vi "TLB Native Dynamic Events ver 0.13a.vi"() -> ()   [LabVIEW 2018]
uses:
  Labview Training Phase 2/Enum Controls/States for Action Engine.ctl
  TLB Type Definitions/State Type Definitions, for 0.26g versions and later 2.ctl
  TLB Type Definitions/Intruction Type Definitions.ctl
  TLB Type Definitions/Encoder cluster.ctl
  Experimental VI's/Archived VI's/MOTOR CONTROL NO PID Type Def.ctl
  Underlying VI's/I2C Master VI/I2C MASTER Type Def.ctl
  TLB Type Definitions/PING CLUSTER.ctl
  <vilib>/Studica/Studica Toolkit/NavX/NavX.lvlib
  <vilib>/Studica/Studica Toolkit/Background/DIO Channel.ctl
  Underlying VI's/NavX VI/navX type def.ctl
  <vilib>/myRIO/Instrument Drivers/Utilities/Utilities.lvlib
  <vilib>/Studica/Studica Toolkit/Background/I2C Channel.ctl
  Underlying VI's/I2C Master VI/I2C_MASTER_WRITE_NEW Type Def.ctl
  <vilib>/userdefined/High Color/IMAQdx.ctl
  Underlying VI's/Webcam FGV Low level ver/State control.ctl
  TLB Type Definitions/Vision cluster.ctl
  <vilib>/NI_Real-Time Target Support.lvlib
  <vilib>/Studica/Studica Toolkit/NavX/TypeDefs/Flags/Z900_navX_Flags_CalibrationStatusTypeDef.ctl
  <vilib>/Studica/Studica Toolkit/NavX/TypeDefs/Flags/Z900_navX_Flags_OpStatusTypeDef.ctl
  <vilib>/Utility/RT CPU Load.ctl
panel:
  out "CPU loads":T1[](array[typedef]) {"ISR (%)" format="%#.2f"; "Idle (%)" format="%#.2f"; "Background (%)" format="%#.2f"; "Normal (%)" format="%#.2f"; "Above Normal (%)" format="%#.2f"; "High (%)" format="%#.2g"; "Timed Structures (%)" format="%#.2g"; "Time Critical (%)" format="%#.2g"; "Total (%)" format="%#.2g"}
  in  "Red LED":bool
  out "Object Center Coordinates":cluster{"x":sgl, "y":sgl}
  out "Object detection cluster":T2
  in  "Mode":enum16{"Ball", "Soap", "Gel", "Pipe", "None"}(ring)
  in  "Latch":bool
  in  "y Stepper value":u8
  out "Arduino Data":T3
  in  "Arduino mode":T4
  out "Detect?":bool
  out "Status":T7 {"OP Status" items=["INITIALIZING", "SELFTEST_IN_PROGRESS", "ERROR", "IMU_AUTOCAL_IN_PROGRESS", "NORMAL"]; "Calibration Status" items=["IMU_CAL_STATE_MASK"=3, "IMU_CAL_STATE_INPROGRESS"=0, "IMU_CAL_STATE_ACCUMULATE"=1, "IMU_CAL_STATE_COMPLETE"=2]}
  out "NavX Readings":T8
  out "TASK ENABLE":bool
  out "Rising Edge":bool
  in  "Green LED":bool
  out "Task Selection":u8
  out "Object detected?":bool
  out "I2C Error":errorcluster
  out "Speed & distance":T9
  out "State Logic":T10=enum."Startup"
  out "elements":T11[](array[typedef])
  in  "STOP TASK":bool
  in  "OK Button":bool
  in  "STOP":bool
  out "error out":errorcluster
  out "Action Queue Items":i32
  out "State Logic Queue Items":i32
  out "Action Queues items":string[](array[string])=["Hardware reset", "Software reset", ""]
  out "Action State":string
  # "TLB FRAMEWORK STATUS"
  # "System Health Status Update"
  # "Test Programme written by Calvin Loke    Dated: 28 Aug 2019\nTest Programme revised by Dr Alex See   Dated 30 Aug 2019\n\nProgramme version:   TLB Native Dynamic Events ver 0.04b.vi"
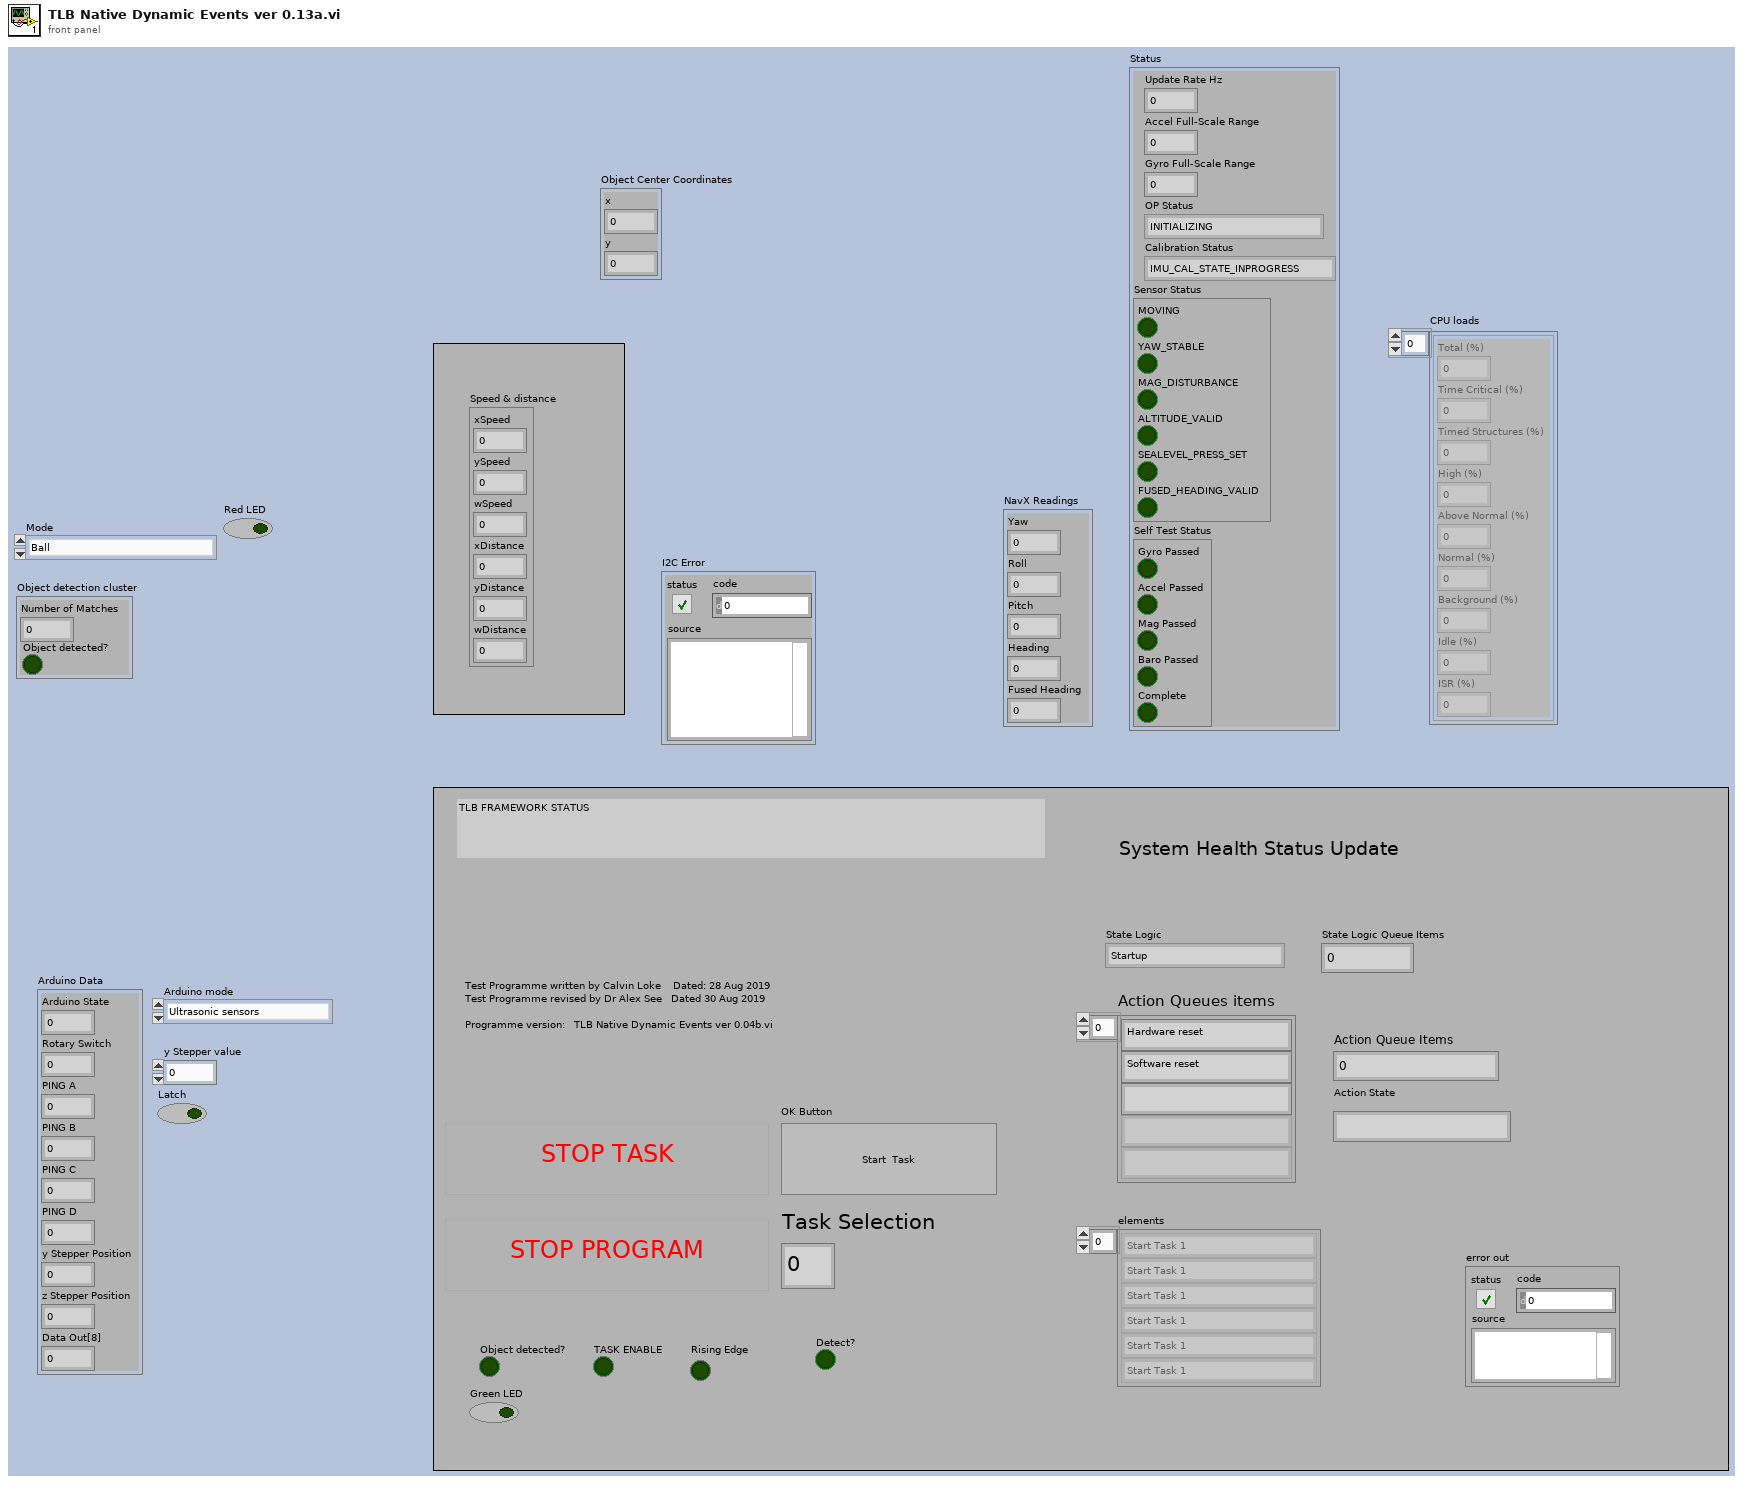
[diagram p1: front panel]
types:
  T1 = typedef "NI_Real-Time Target Support.lvlib/RT CPU Load.ctl" = cluster{"Total (%)":dbl, "Time Critical (%)":dbl, "Timed Structures (%)":dbl, "High (%)":dbl, "Above Normal (%)":dbl, "Normal (%)":dbl, "Background (%)":dbl, "Idle (%)":dbl, "ISR (%)":dbl}
  T2 = cluster{"Number of Matches":i32, "Object detected?":bool}
  T3 = cluster{"Arduino State":u8, "Rotary Switch":u8, "PING A":u8, "PING B":u8, "PING C":u8, "PING D":u8, "y Stepper Position":u8, "z Stepper Position":u8, "Data Out[8]":u8}
  T4 = typedef "I2C_MASTER_WRITE_NEW Type Def.ctl" = enum16{"Ultrasonic sensors", "Stepper origin", "zStepper 13.3k", "zStepper 13k", "zStepper 12k", "zStepper 11k", "zStepper 10k", "zStepper 9k", "zStepper 8k", "zStepper 7k", "zStepper 6k", "zStepper 5k", "zStepper 4k", "zStepper 3k", "zStepper 2k", "zStepper 1k", "zStepper 900", "zStepper 800", "zStepper 700", "zStepper 600", "zStepper 500", "zStepper 400", "zStepper 300", "zStepper 200", "zStepper 100", "zStepper 0", "yStepper control", "Open Claw", "Close Claw", "Soft Reset"}
  T5 = typedef "NavX.lvlib/Z900_navX_Flags_OpStatusTypeDef.ctl" = u8
  T6 = typedef "NavX.lvlib/Z900_navX_Flags_CalibrationStatusTypeDef.ctl" = u8
  T7 = cluster{"Update Rate Hz":u8, "Accel Full-Scale Range":u8, "Gyro Full-Scale Range":u16, "OP Status":T5, "Calibration Status":T6, "Sensor Status":cluster{"MOVING":bool, "YAW_STABLE":bool, "MAG_DISTURBANCE":bool, "ALTITUDE_VALID":bool, "SEALEVEL_PRESS_SET":bool, "FUSED_HEADING_VALID":bool}, "Self Test Status":cluster{"Gyro Passed":bool, "Accel Passed":bool, "Mag Passed":bool, "Baro Passed":bool, "Complete":bool}}
  T8 = cluster{"Yaw":dbl, "Roll":dbl, "Pitch":dbl, "Heading":dbl, "Fused Heading":dbl}
  T9 = cluster{"xSpeed":dbl, "ySpeed":dbl, "wSpeed":dbl, "xDistance":dbl, "yDistance":dbl, "wDistance":dbl}
  T10 = typedef "State Type Definitions, for 0.26g versions and later 2.ctl" = enum16{"None", "Startup", "Move to Angle", "True Stop", "Idle", "Shutdown", "Task 1A", "Task 1B", "Task 2:Raise Arm", "Task 2:Sensor Mode", "Task 2:Reverse Mode", "Task 3", "Task 4_A", "Task 4_B", "Task 4_C", "Task 4_D", "Task 5A", "Task 5B", "Task 5C", "Task 5D", "Task 5E: POSITION ARM", "Task 5F: ARM GRAB HEIGHT", "Task 5G: CLOSE CLAW", "Task 5H: RAISE ARM", "Task 6_A", "Task 6_B", "Task 7", "Task 8A: RAISE ARM", "Task 8B: MOVE TO BOX", "Task 8C: CAM BURST", "Task 8D: PROCESS IMAGE", "Task 8E: ROBOT ADJUST", "Task 8F: CAM BURST 2", "Task 8G: PROCESS IMAGE 2", "Task 8H: ARM ADJUST", "Task 8I: ARM GRAB HEIGHT", "Task 8J: CLOSE CLAW", "Task 8K: RAISE MY SWORD", "Task 9A: Raise Arm", "Task 9B: Rotate to Angle", "Task 9C: Detect Box", "Task 9D: MOVE FORWARD", "Task 9E: MOVE LEFT", "Task 9F: SCAN BOX", "Task 9G: MOVE RIGHT", "Task 9H: SCAN BOX 2", "Task 9I: ROTATE 90 CW", "Task 9J: FORWARD", "Task 9K: MOVE RIGHT", "Task 9L: SCAN BOX 3", "Task 9M: MOVE RIGHT", "Task 9N: SCAN BOX 4", "PENIS", "PENIS 2", "PENIS 3", "Task 9R: PROCESS COLOUR", "Task A1: Task 9 Open cam", "Task A2: Task 9 Move Arm", "Task A3: Task 9 Set Timer", "Task A4: Tasl 9 Capture images", "Task A5: Task 9 Close camera", "Task A6: Process Colour", "Task A7: Dispose Camera Buffer"}
  T11 = typedef "Intruction Type Definitions.ctl" = enum16{"None", "Start Task 1", "Start Task 2", "Start Task 3", "Start Task 4", "Start Task 5", "Start Task 6", "Start Task 7", "Start Task 8 - BALL", "Start Task 8 - Gel", "Start Task 8 - Pipe", "Start Task 8 - Soap", "Start Task 9", "Start Task A", "Start Task B", "Exit"}
  T12 = typedef "States for Action Engine.ctl" = enum16{"Initialize", "Write", "Read"}
  T13 = typedef "DIO Channel.ctl" = enum16{"Not Connected", "A/DIO1", "A/DIO2", "A/DIO3", "A/DIO4", "A/DIO5", "A/DIO6", "A/DIO7", "A/DIO13", "B/DIO1", "B/DIO2", "B/DIO3", "B/DIO4", "B/DIO5", "B/DIO6", "B/DIO7", "B/DIO13", "C/DIO0", "C/DIO1", "C/DIO2", "C/DIO3", "C/DIO4", "C/DIO5", "C/DIO6", "C/DIO7"}
  T14 = typedef "Vision cluster.ctl" = cluster{"Recognized Object":bool, "Object X coordinate":dbl, "Object Y coordinate":dbl}
  T15 = typedef "PING CLUSTER.ctl" = cluster{"PING_A":u8, "PING_B":u8, "PING_C":u8, "PING_D":u8}
  T16 = typedef "Encoder cluster.ctl" = cluster{"xDistance":dbl, "yDistance":dbl, "wDistance":dbl}
  T17 = typedef "I2C Channel.ctl" = enum16{"Not Connected", "A", "B"}
  T18 = typedef "navX type def.ctl" = enum16{"Get i2C reference", "Read Values", "Zero Yaw"}
  T19 = typedef "State Type Definitions.ctl" = enum16{"None", "Startup", "Move to Angle", "True Stop", "Idle", "Shutdown", "Task 1", "Task 2:Raise Arm", "Task 2:Sensor Mode", "Task 2:Reverse Mode", "Task 3", "Task 4_A", "Task 4_B", "Task 4_C", "Task 4_D", "Task 5A: ARM CAM HEIGHT", "Task 5B: MOVE TO BOX", "Task 5C: CAM BURST", "Task 5D: PROCESS IMAGE", "Task 5E: POSITION ARM", "Task 5F: ARM GRAB HEIGHT", "Task 5G: CLOSE CLAW", "Task 5H: RAISE ARM", "Task 6_A", "Task 6_B", "Task 7", "Task 8A: RAISE ARM", "Task 8B: MOVE TO BOX", "Task 8C: CAM BURST", "Task 8D: PROCESS IMAGE", "Task 8E: ROBOT ADJUST", "Task 8F: CAM BURST 2", "Task 8G: PROCESS IMAGE 2", "Task 8H: ARM ADJUST", "Task 8I: ARM GRAB HEIGHT", "Task 8J: CLOSE CLAW", "Task 8K: RAISE MY SWORD", "Task 9A: Raise Arm", "Task 9B: Rotate to Angle", "Task 9C: Detect Box", "Task 9D: MOVE FORWARD", "Task 9E: MOVE LEFT", "Task 9F: SCAN IMAGE", "Task 9G: PROCESS COLOUR", "Task 9H: MOVE RIGHT", "Task 9I: SCAN IMAGE", "Task 9J: PROCESS COLOUR", "Task 9K: ROTATE 90 CW", "Task 9L: MOVE FORWARD", "Task 9M: MOVE RIGHT", "Task 9N: SCAN IMAGE", "Task 9O: PROCESS COLOUR", "Task 9P: MOVE RIGHT", "Task 9Q: SCAN IMAGE", "Task 9R: PROCESS COLOUR"}
  T20 = typedef "State Type Definitions.ctl" = enum16{"None", "Startup", "Move to Angle", "True Stop", "Idle", "Shutdown", "Task 1", "Task 2", "Task 3", "Task 4_A", "Task 4_B", "Task 4_C", "Task 5", "Task 6", "Task 7", "Task 8", "Task 9", "Task A", "Task B"}
  T21 = typedef "MOTOR CONTROL NO PID Type Def.ctl" = enum16{"Init", "Front Back", "Left Right", "Rotate", "Stop", "Latch"}
  T22 = typedef "State control.ctl" = enum16{"Initialise", "Start camera", "Continuous Acquisition ", "Stop camera", "Dispose all"}
  T23 = typedef "IMAQdx.ctl" = refnum<k21>
  T24 = cluster{"DIO Channel":T13, "FPGA VI Reference Out":refnum<k20>}
  T25 = cluster{"I2C Ref Out":cluster{"I2C Channel":T17, "FPGA VI Reference Out":refnum<k20>}, "Connected":bool, "Slave Address (7-bit)":u8, "Registry":u8[]}
  T26 = typedef "IMAQ Image.ctl" = refnum<image>
  T27 = typedef "I2C MASTER Type Def.ctl" = enum16{"Last State", "Mode 0", "Mode 1", "Mode 2", "Mode 3", "Mode 4", "Mode 5", "Mode 6", "Mode 7", "Mode 8", "Mode 9", "Mode 10"}
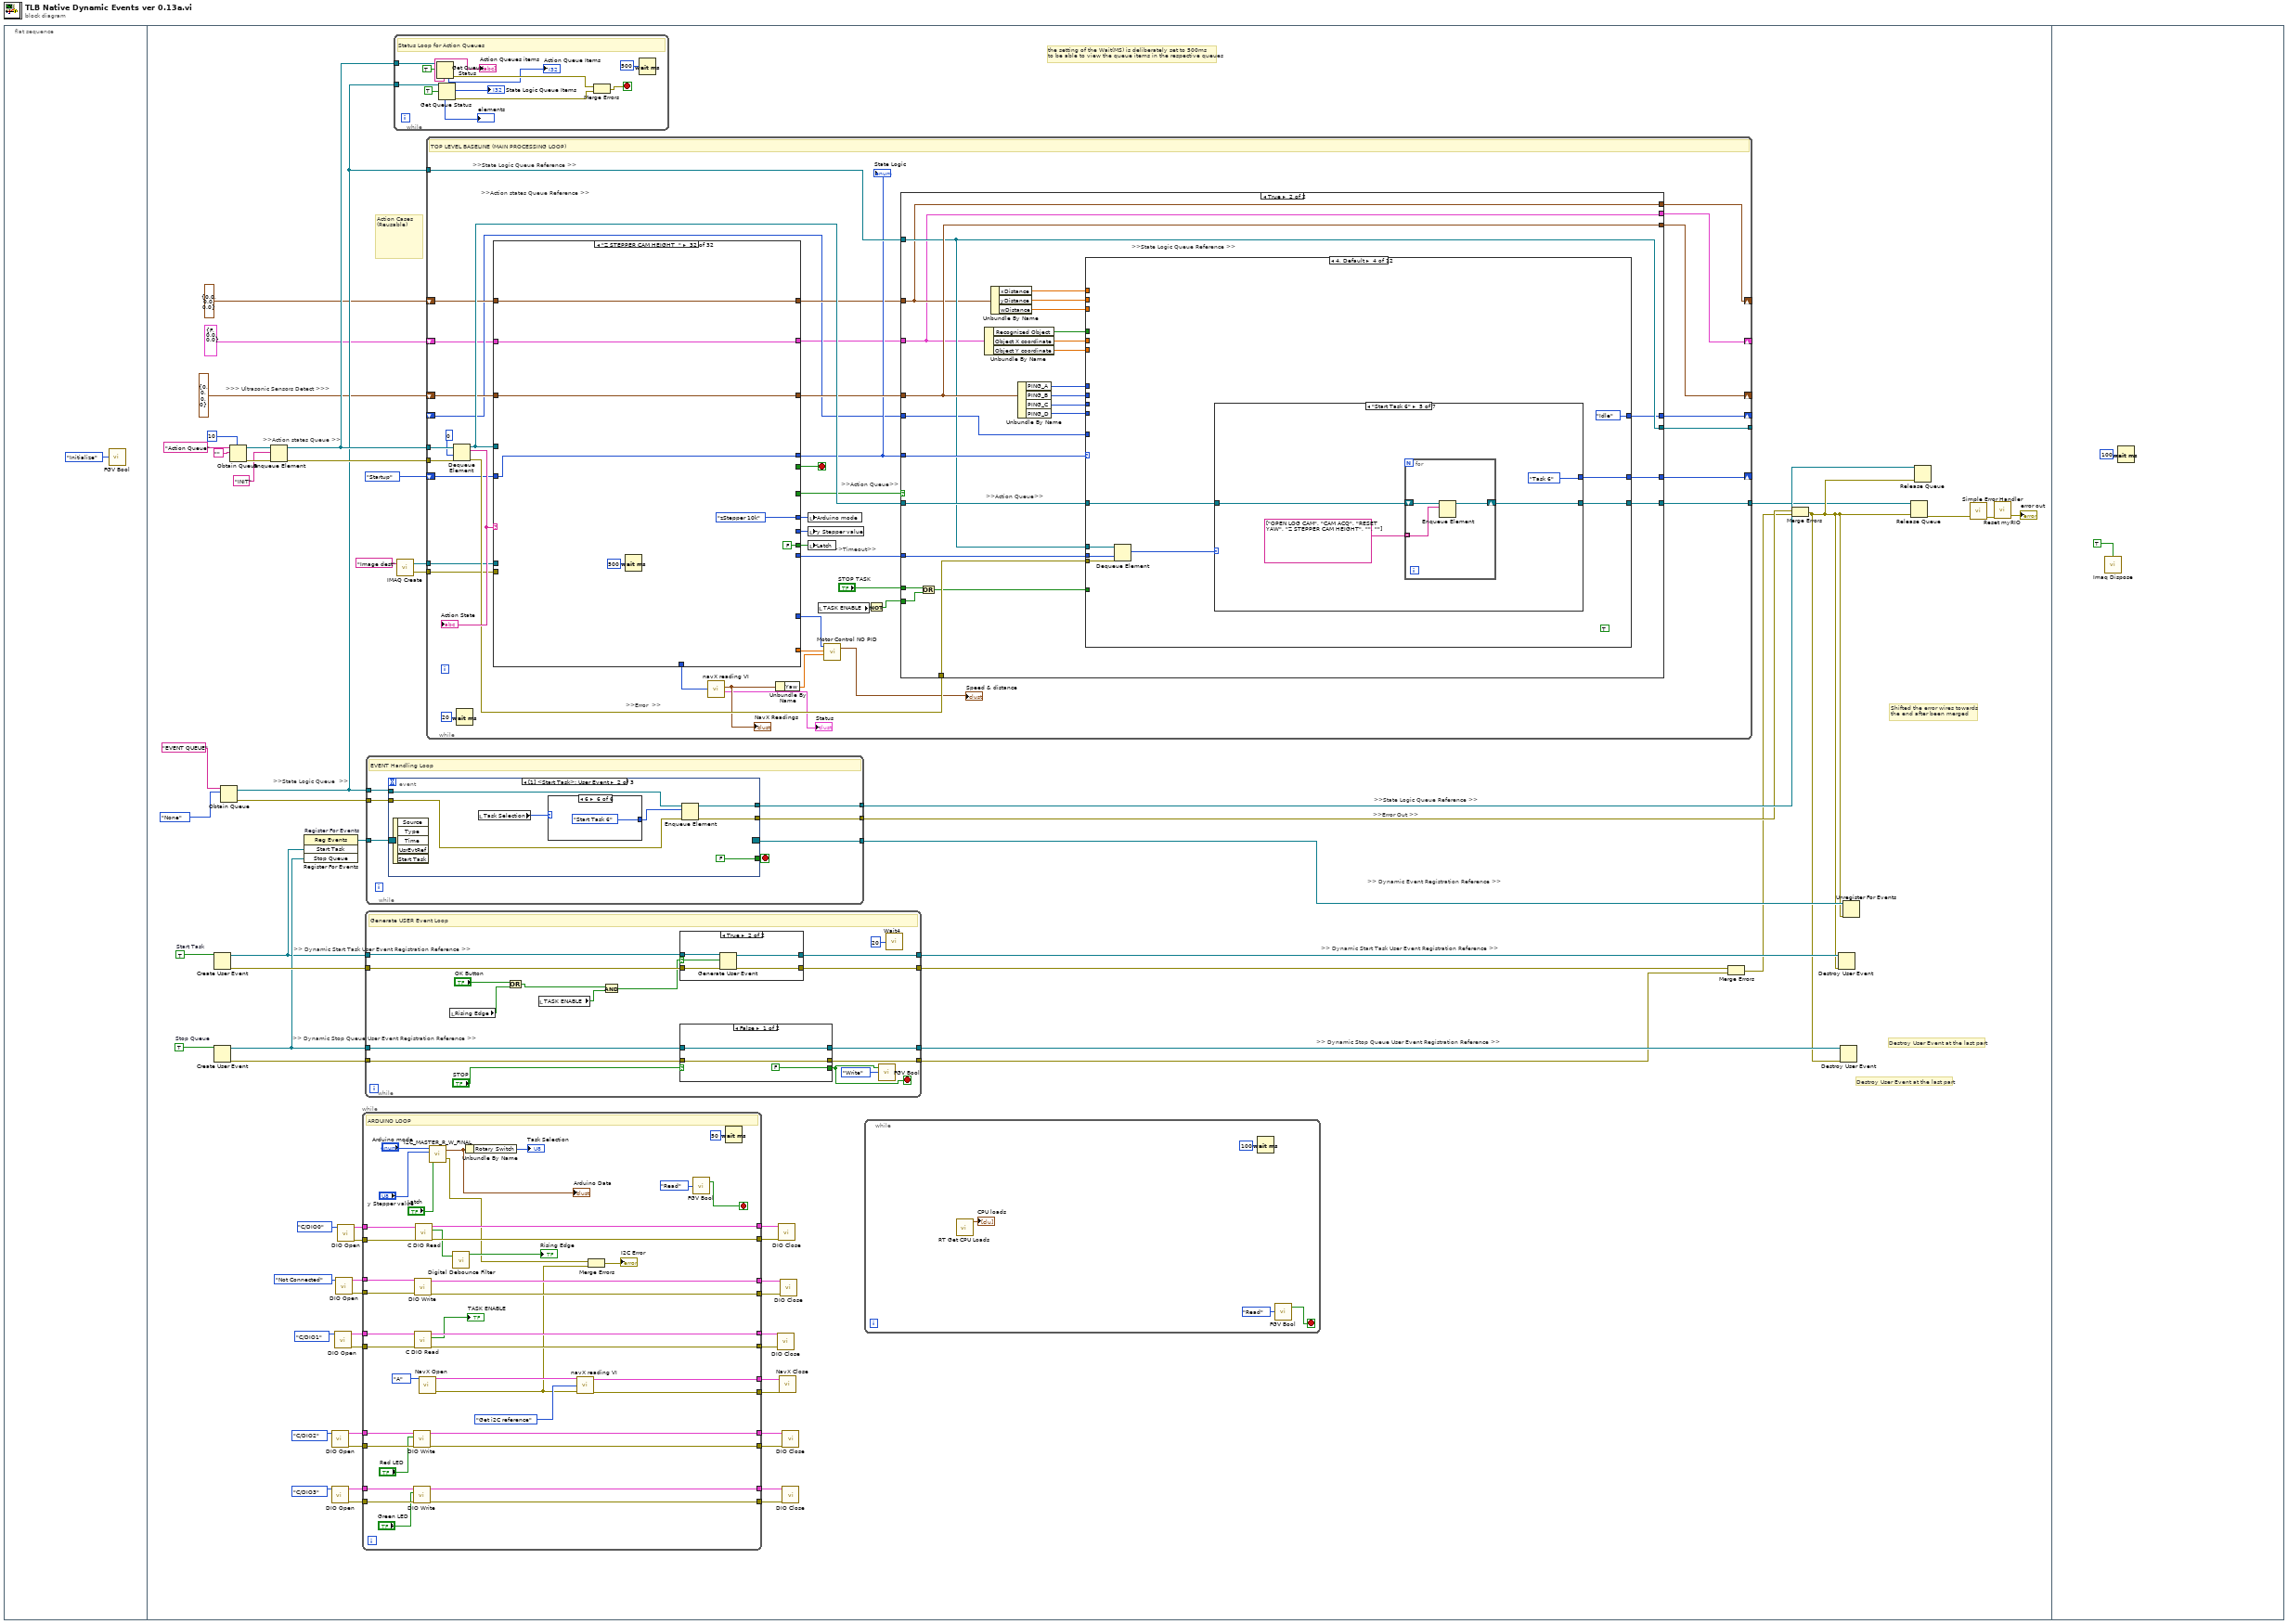
[diagram p0: block diagram]
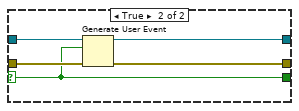
[diagram p2: hidden frame]
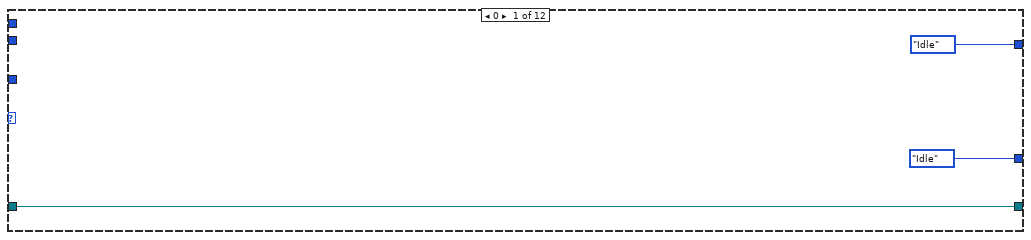
[diagram p5: hidden frame]
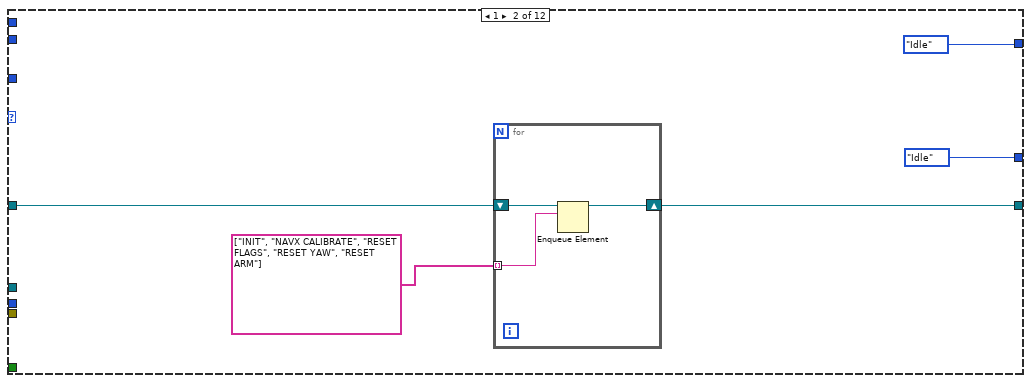
[diagram p6: hidden frame]
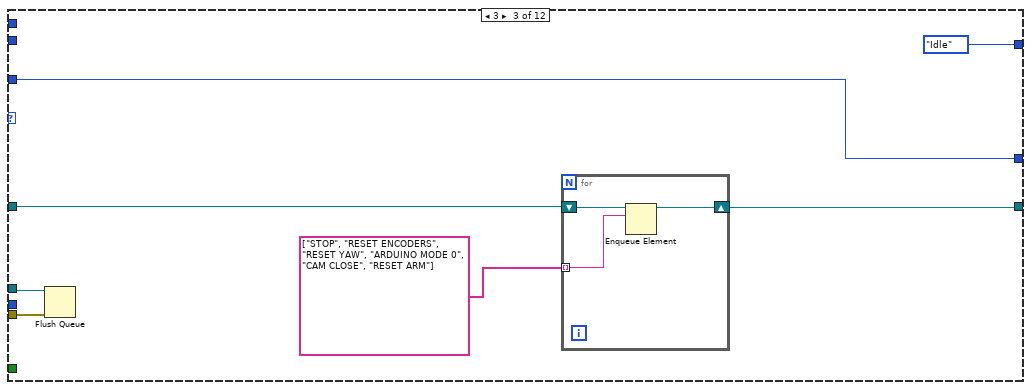
[diagram p7: hidden frame]
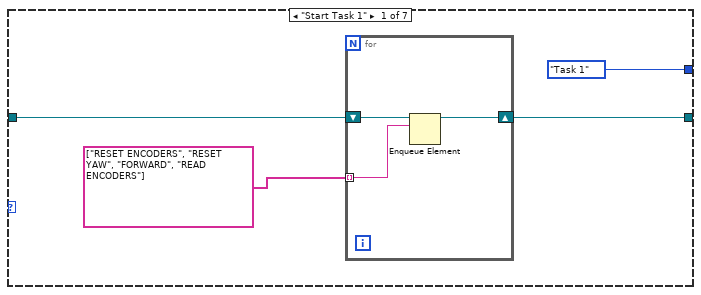
[diagram p8: hidden frame]
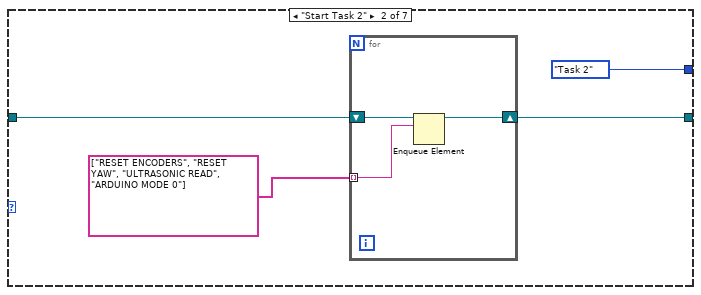
[diagram p9: hidden frame]
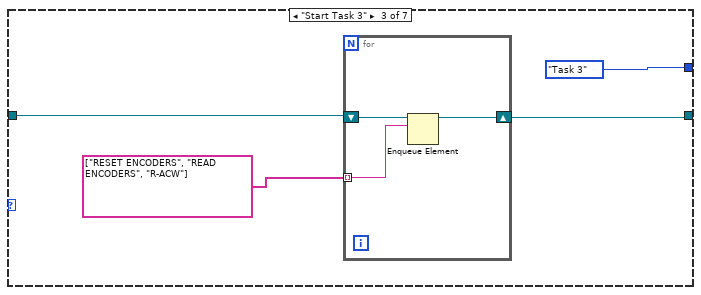
[diagram p10: hidden frame]
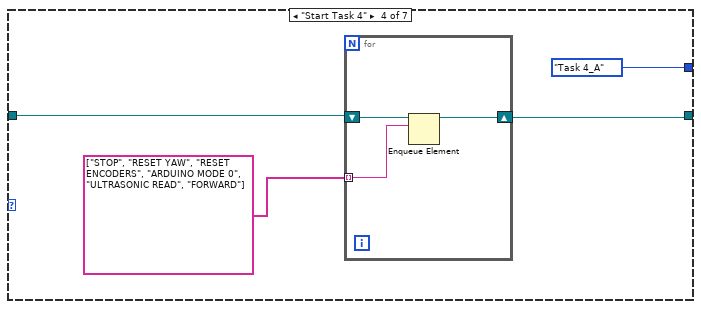
[diagram p11: hidden frame]
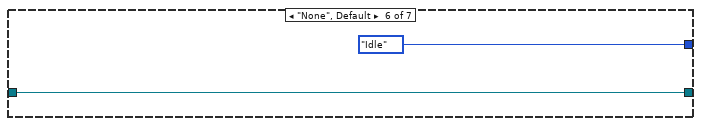
[diagram p12: hidden frame]
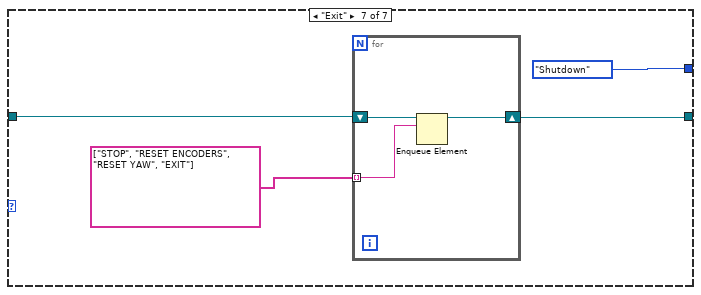
[diagram p13: hidden frame]
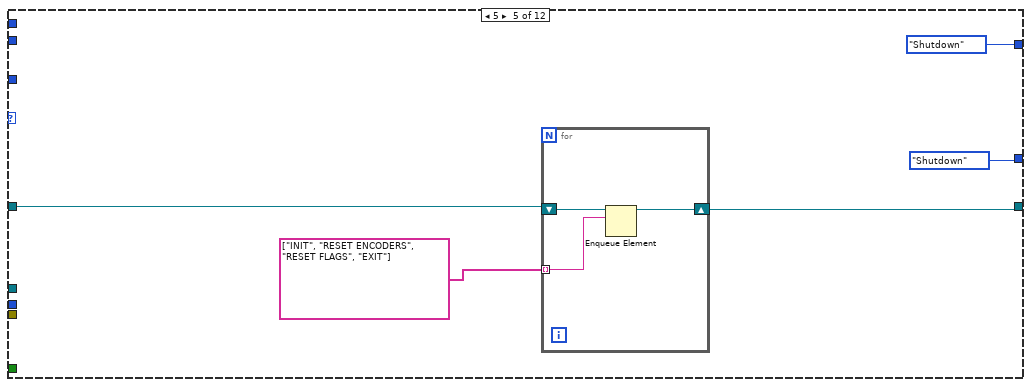
[diagram p14: hidden frame]
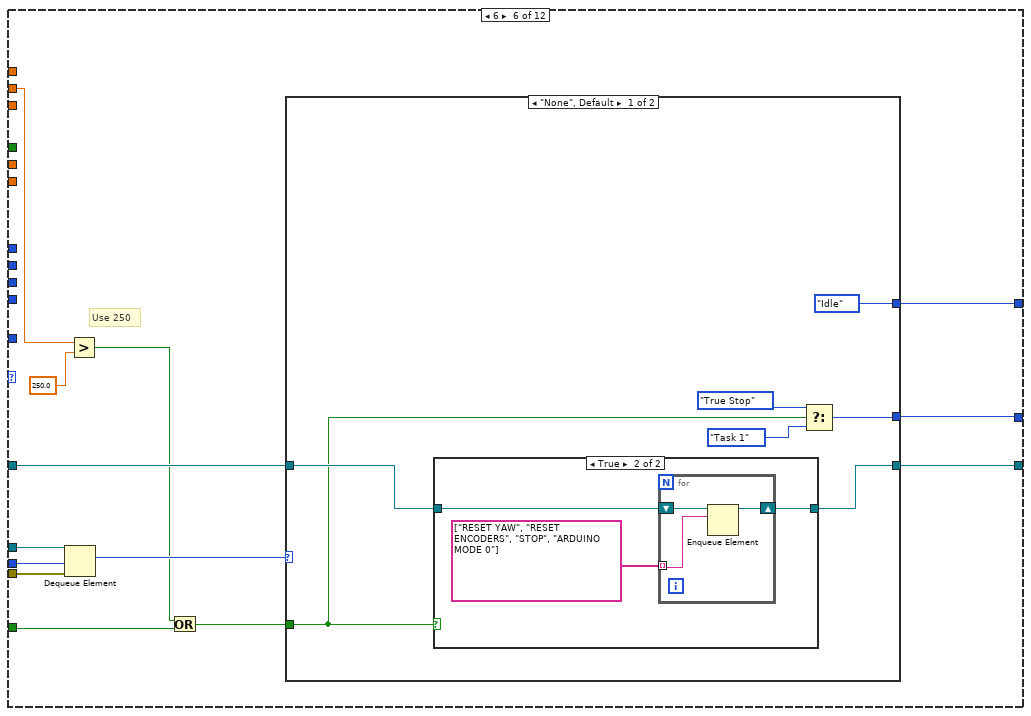
[diagram p15: hidden frame]
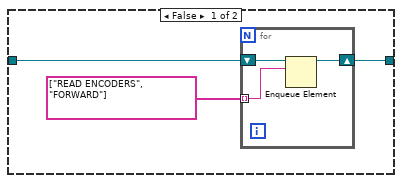
[diagram p16: hidden frame]
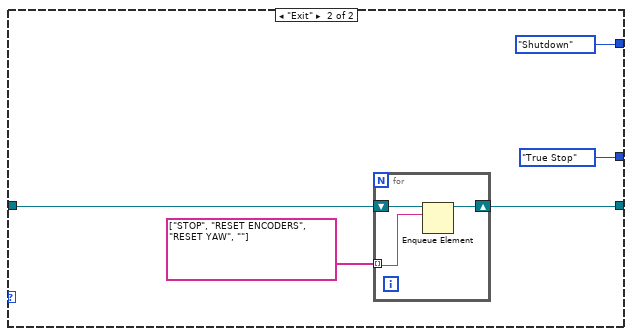
[diagram p17: hidden frame]
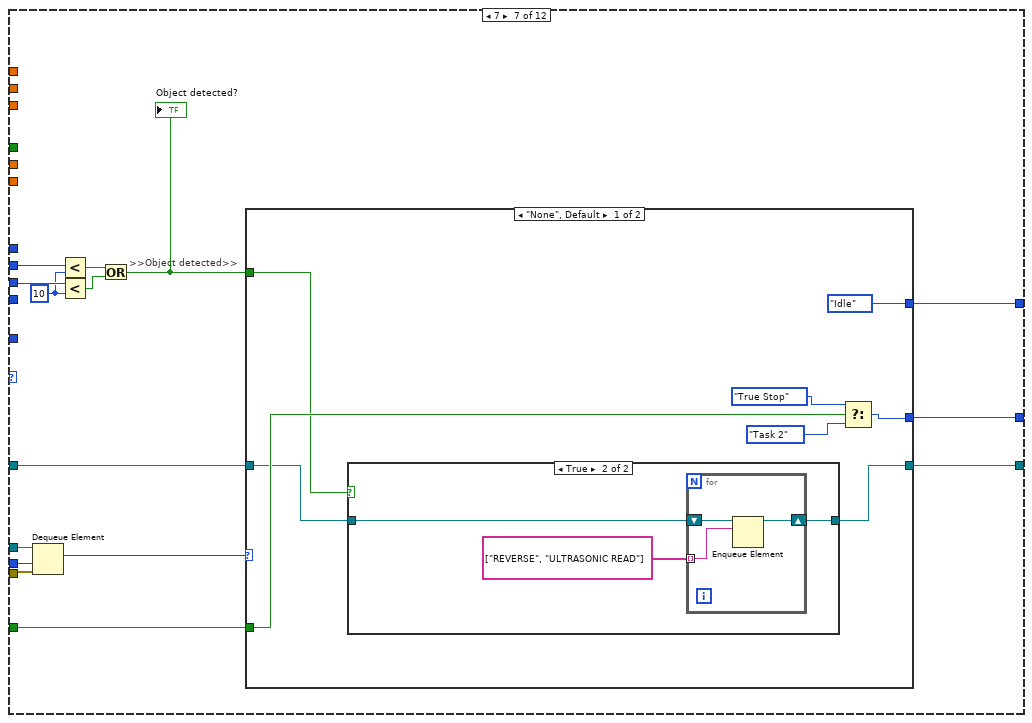
[diagram p18: hidden frame]
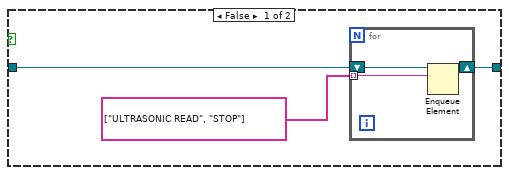
[diagram p19: hidden frame]
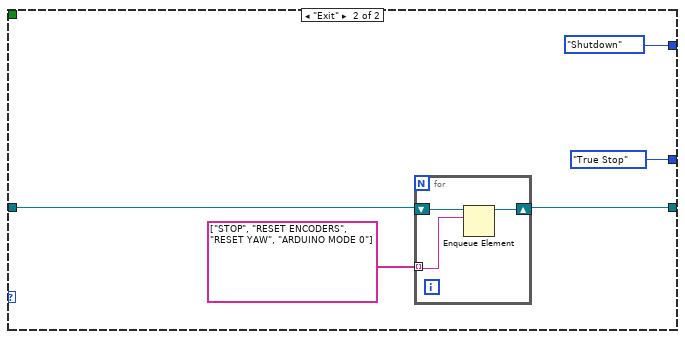
[diagram p20: hidden frame]
diagram:
  n1 = flat-sequence {
    frame #0 {
      n2 = call "FGV Bool.vi"("Init/Read/Write State"=States_for_Action_Engine."Initialize") -> ()  [unwired: 2 in, 2 out]
    }
    frame #1 {
      w67 = TRUE  # Stop Queue
      w66 = TRUE  # Start Task
      # ">>> Ultrasonic Sensors Detect >>>"
      # "the setting of the Wait(MS) is deliberately set to 500ms\nto be able to view the queue items in the respective queues"
      # "Action Cases\n(Reusable)"
      # ">>Error Out >>"
      # ">> Dynamic Stop Queue User Event Registration Reference >>"
      # ">> Dynamic Start Task User Event Registration Reference >>"
      # ">> Dynamic Stop Queue User Event Registration Reference >>"
      # ">> Dynamic Start Task User Event Registration Reference >>"
      # ">> Dynamic Event Registration Reference >>"
      # ">>Action states Queue >>"
      # ">>State Logic Queue  >>"
      # ">>State Logic Queue Reference >>"
      # "Destroy User Event at the last part"
      # "Destroy User Event at the last part"
      # "Shifted the error wires towards\nthe end after been merged"
      n3 = Create User Event(user event datatype=w66) -> (user event=w58:refnum<user-event>, error out=w63:errorcluster)  [unwired: 1 in]
      n4 = Create User Event(user event datatype=w67) -> (user event=w59:refnum<user-event>, error out=w62:errorcluster)  [unwired: 1 in]
      n5 = Obtain Queue(name (unnamed)="EVENT QUEUE", element data type=Intruction_Type_Definitions."None" ("Enum")) -> (queue out=w44:refnum<queue>, error out=w50:errorcluster)  [unwired: 3 in, 1 out]
      n6 = Obtain Queue(max queue size (-1, unlimited)=10, name (unnamed)="Action Queue", element data type="") -> (queue out=w53:refnum<queue>, error out=w49:errorcluster)  [unwired: 2 in, 1 out]
      n7 = Enqueue Element(queue=w53, element="INIT", error in (no error)=w49) -> (queue out=w45:refnum<queue>, error out=w48:errorcluster)  [unwired: 1 in, 1 out]
      n8 = register-events "Register For Events"(w58, w59) -> (reference out=w57:refnum<event-registration>)  [unwired: 2 in, 1 out]
      n9 = call <vilib>:"DIO Open.vi"("DIO Channel"=DIO_Channel."C/DIO2") -> ("error out"=w9:errorcluster, "DIO Info Out"=w10:T24)  [unwired: 9 in]
      n10 = call <vilib>:"DIO Open.vi"("DIO Channel"=DIO_Channel."C/DIO3") -> ("error out"=w4:errorcluster, "DIO Info Out"=w5:T24)  [unwired: 9 in]
      n11 = call <vilib>:"DIO Open.vi"("DIO Channel"=DIO_Channel."C/DIO1") -> ("error out"=w22:errorcluster, "DIO Info Out"=w23:T24)  [unwired: 9 in]
      n12 = call <vilib>:"DIO Open.vi"("DIO Channel"=DIO_Channel."Not Connected") -> ("error out"=w27:errorcluster, "DIO Info Out"=w29:T24)  [unwired: 9 in]
      n13 = call <vilib>:"DIO Open.vi"("DIO Channel"=DIO_Channel."C/DIO0") -> ("error out"=w32:errorcluster, "DIO Info Out"=w35:T24)  [unwired: 9 in]
      n14 = while {
        tunnel: w35 -> [w108]
        tunnel: [w107] -> w33
        tunnel: w32 -> [w106]
        tunnel: [w105] -> w31
        tunnel: w29 -> [w101]
        tunnel: [w100] -> w28
        tunnel: w27 -> [w99]
        tunnel: [w98] -> w26
        tunnel: [w97] -> w24
        tunnel: w23 -> [w96]
        tunnel: w22 -> [w95]
        tunnel: [w94] -> w21
        tunnel: [w91] -> w20
        tunnel: [w90] -> w19
        tunnel: w10 -> [w81]
        tunnel: w9 -> [w80]
        tunnel: [w79] -> w8
        tunnel: [w78] -> w7
        tunnel: w5 -> [w76]
        tunnel: w4 -> [w75]
        tunnel: [w74] -> w3
        tunnel: [w73] -> w2
        stop <- w111 stop-if-true
        # "ARDUINO LOOP"
        n15 = call <vilib>:"DIO Write.vi"("error in (no error)"=w80, "Input"="Red LED", "DIO Info In"=w81) -> ("error out"=w78:errorcluster, "DIO Info Out"=w79:T24)  [unwired: 7 in]
        n16 = call <vilib>:"DIO Write.vi"("error in (no error)"=w75, "Input"="Green LED", "DIO Info In"=w76) -> ("error out"=w73:errorcluster, "DIO Info Out"=w74:T24)  [unwired: 7 in]
        n17 = call <vilib>:"DIO Write.vi"("error in (no error)"=w99, "DIO Info In"=w101) -> ("error out"=w98:errorcluster, "DIO Info Out"=w100:T24)  [unwired: 8 in]
        n18 = call <vilib>:"C DIO Read.vi"("error in (no error)"=w95, "DIO Info In in"=w96) -> ("error out"=w94:errorcluster, "IN"=→"TASK ENABLE":bool, "DIO Info In out"=w97:T24)  [unwired: 7 in]
        n19 = call <vilib>:"C DIO Read.vi"("error in (no error)"=w106, "DIO Info In in"=w108) -> ("error out"=w105:errorcluster, "IN"=w103:bool, "DIO Info In out"=w107:T24)  [unwired: 7 in]
        n20 = call <vilib>:"NavX Open.vi"("I2C Channel"=I2C_Channel."A") -> ("error out"=w88:errorcluster, "NavX Info"=w92:T25)  [unwired: 9 in]
        n21 = call "I2C_MASTER_R_W_FINAL.vi"("Latch"="Latch", "y Stepper value"="y Stepper value", "Arduino mode"="Arduino mode") -> ("error out"=w85:errorcluster, "Arduino Data"=w84:T3)  [unwired: 1 in]
        "Arduino Data" <- w84
        n22 = call "Digital Debounce Filter.vi"("Boolean input"=w103) -> ("Rising Edge"=→"Rising Edge":bool)  [unwired: 1 in, 2 out]
        n23 = Unbundle By Name(w84) -> ("Rotary Switch"=→"Task Selection":u8)
        n24 = call "navX reading VI.vi"("NavX Info In"=w92, "Mode"=navX_type_def."Get i2C reference", "error in (no error)"=w88) -> ("NavX Info Out"=w91:T25, "Error Out"=w90:errorcluster)  [unwired: 2 out]
        n25 = Merge Errors(w85, w88) -> (→"I2C Error":errorcluster)
        n26 = call "FGV Bool.vi"("Init/Read/Write State"=States_for_Action_Engine."Read") -> ("Output node"=w111:bool)  [unwired: 2 in, 1 out]
        n27 = Wait (ms)(milliseconds to wait=u32 50) -> ()  [unwired: 1 out]
      }
      n28 = while {
        tunnel: w58 -> [w141]
        tunnel: w59 -> [w140]
        tunnel: [w139] -> w65
        tunnel: [w138] -> w64
        tunnel: w63 -> [w137]
        tunnel: [w136] -> w61
        tunnel: w62 -> [w135]
        tunnel: [w134] -> w60
        stop <- w132 stop-if-true
        # "Generate USER Event Loop"
        n29 = local read "Rising Edge"() -> (w128:bool)
        n30 = Or(x="OK Button", y=w128) -> (x .or. y?=w127:bool)
        n31 = local read "TASK ENABLE"() -> (w126:bool)
        n32 = And(x=w127, y=w126) -> (x .and. y?=w125:bool)
        n33 = case shown="True" w125 {
          selector: w125 -> [_ w152]
          tunnel: w141 -> [w151 w156]
          tunnel: [w151 w155] -> w138
          tunnel: w137 -> [w150 w154]
          tunnel: [w150 w153] -> w136
          frame False {
          }
          frame True {
            n34 = Generate User Event(user event=w156, event data cluster=w152, error in=w154) -> (user event out=w155:refnum<user-event>, error out=w153:errorcluster)  [unwired: 1 in]
          }
        }
        n35 = case shown="False" "STOP" {
          selector: "STOP" -> [_ w145]
          tunnel: w140 -> [w144 w149]
          tunnel: [w144 w148] -> w139
          tunnel: w135 -> [w143 w147]
          tunnel: [w143 w146] -> w134
          tunnel: [FALSE w145] -> w132
          frame False {
          }
          frame True {
            n36 = Generate User Event(user event=w149, event data cluster=w145, error in=w147) -> (user event out=w148:refnum<user-event>, error out=w146:errorcluster)  [unwired: 1 in]
          }
        }
        n37 = call "FGV Bool.vi"("Init/Read/Write State"=States_for_Action_Engine."Write", "Input Node"=w132) -> ()  [unwired: 1 in, 2 out]
        n38 = call "Wait4"("Count(uSec)"=u32 20) -> ()  [unwired: 1 out]
      }
      n39 = while {
        tunnel: w57 -> [w860]
        tunnel: [w859] -> w56
        tunnel: w44 -> [w857]
        tunnel: [w856] -> w55
        tunnel: w50 -> [w855]
        tunnel: [w854] -> w47
        stop <- w858 stop-if-true
        # "EVENT Handling Loop"
        n40 = event shown="[1] <Start Task>: User Event" {
          selector: w860 -> [_ _ _]
          dyn-events: [_ _ _] -> w859
          timeout: _ -> [_ _ _]
          tunnel: [FALSE FALSE w885] -> w858
          tunnel: w857 -> [w865 w872 w883]
          tunnel: [w864 w871 w884] -> w856
          tunnel: w855 -> [w863 w870 w882]
          tunnel: [w862 w869 w881] -> w854
          event Timeout {
            n41 = event-data() -> ()  [unwired: 1 in, 3 out]
            n42 = Enqueue Element(queue=w865, element=Intruction_Type_Definitions."None" ("Enum"), error in (no error)=w863) -> (queue out=w864:refnum<queue>, error out=w862:errorcluster)  [unwired: 1 in, 1 out]
          }
          event User Event {
            n43 = event-data() -> ()  [unwired: 1 in, 5 out]
            n44 = local read "Task Selection"() -> (w867:u8)
            n45 = case shown="6" w867 {
              tunnel: [Intruction_Type_Definitions."None" ("Enum") Intruction_Type_Definitions."Start Task 1" ("Enum") Intruction_Type_Definitions."Start Task 2" ("Enum") Intruction_Type_Definitions."Start Task 3" ("Enum") Intruction_Type_Definitions."Start Task 4" ("Enum") Intruction_Type_Definitions."Start Task 6" ("Enum")] -> w868
              frame 0, Default {
              }
              frame 1 {
              }
              frame 2 {
              }
              frame 3 {
              }
              frame 4 {
              }
              frame 6 {
              }
            }
            n46 = Enqueue Element(queue=w872, element=w868, error in (no error)=w870) -> (queue out=w871:refnum<queue>, error out=w869:errorcluster)  [unwired: 1 in, 1 out]
          }
          event User Event {
            n47 = event-data() -> ("Stop Queue"=w885:bool)  [unwired: 1 in, 4 out]
            n48 = Enqueue Element At Opposite End(queue=w883, element=Intruction_Type_Definitions."Exit" ("Enum"), error in (no error)=w882) -> (queue out=w884:refnum<queue>, error out=w881:errorcluster)  [unwired: 1 in, 1 out]
          }
        }
      }
      n49 = while {
        tunnel: w45 -> [w122]
        tunnel: w44 -> [w119]
        stop <- w116 stop-if-true
        # "Status Loop for Action Queues"
        n50 = Get Queue Status(queue=w122, return elements? (F)=TRUE) -> (error out=w118:errorcluster, # elements in queue=→"Action Queue Items":i32, elements=→"Action Queues items":string[])  [unwired: 1 in, 5 out]
        n51 = Get Queue Status(queue=w119, return elements? (F)=TRUE) -> (# pending remove=→"State Logic Queue Items":i32, error out=w117:errorcluster, elements=→"elements":T11[])  [unwired: 1 in, 5 out]
        n52 = Merge Errors(w118, w117) -> (w116:errorcluster)
        n53 = Wait (ms)(milliseconds to wait=u32 500) -> ()  [unwired: 1 out]
      }
      n54 = call "IMAQ Create"("Image Name"="Image dest") -> ("New Image"=w14:T26, "error out"=w13:errorcluster)  [unwired: 4 in]
      n55 = while {
        tunnel: w44 -> [w186]
        tunnel: w45 -> [w198]
        tunnel: w48 -> [w196]
        tunnel: [w195] -> _
        tunnel: [w194] -> w38
        shift-right: [w187] -> _
        shift-left: T15 {"PING_A"=0, "PING_B"=0, "PING_C"=0, "PING_D"=0} -> [w189]
        shift-right: [w180] -> _
        shift-left: State_Type_Definitions,_for_0.26g_versions_and_later_2."Startup" ("Enum") -> [w183]
        shift-right: [w176] -> _
        shift-left: T16 {"xDistance"=0.0, "yDistance"=0.0, "wDistance"=0.0} -> [w178]
        shift-right: [w170] -> _
        shift-left: _ -> [w169]
        tunnel: w14 -> [w161]
        tunnel: w13 -> [w160]
        shift-right: [w157] -> _
        shift-left: T14 {"Recognized Object"=FALSE, "Object X coordinate"=0.0, "Object Y coordinate"=0.0} -> [w159]
        stop <- w185 stop-if-true
        # ">>Error  >>"
        # ">>Action Queue>>"
        # ">>Timeout>>"
        # ">>Action states Queue Reference >>"
        # ">>State Logic Queue Reference >>"
        # "TOP LEVEL BASELINE (MAIN PROCESSING LOOP)"
        n56 = Dequeue Element(queue=w198, timeout in ms (-1)=0, error in (no error)=w196) -> (queue out=w190:refnum<queue>, element=w197:string, error out=w191:errorcluster)  [unwired: 1 out]
        "Action State" <- w197
        n57 = Wait (ms)(milliseconds to wait=u32 20) -> ()  [unwired: 1 out]
        n58 = case shown="\"Z STEPPER CAM HEIGHT  \"" w197 {
          tunnel: [_ _ _ _ _ _ _ _ _ _ _ _ _ _ _ _ 0 w738 _ _ _ _ _ _ _ _ _ _ _ _ _ _] -> w193
          tunnel: w190 -> [_ _ _ _ _ _ _ _ _ _ _ _ _ _ _ _ _ _ _ _ _ _ _ _ _ _ _ _ _ _ _ _]
          tunnel: w189 -> [w622 w627 w634 w640 w646 w651 w658 w665 w671 w674 w686 w698 w702 w712 w717 w721 w729 w739 w744 w749 w767 w775 w778 w783 w794 w805 w821 w831 w834 w839 w844 w851]
          tunnel: [w622 w627 w634 w640 w646 w651 w658 w665 w671 w674 w686 w699 w702 w713 w717 w721 w729 w739 w744 w749 w766 w775 w778 w783 w794 w805 w821 w831 w834 w839 w844 w851] -> w188
          tunnel: [TRUE TRUE _ _ _ _ _ _ _ _ _ _ _ _ _ _ _ _ _ _ _ _ _ _ _ _ _ _ _ _ _ _] -> w185
          tunnel: w183 -> [w620 w625 w633 w639 w645 w650 w657 w664 w670 w673 w685 w697 w701 w711 w716 w720 w726 w736 w743 w748 w765 w774 w776 w782 w788 w799 w820 w826 w833 w838 w842 w850]
          tunnel: [_ _ _ _ _ _ _ _ _ _ _ _ _ _ _ _ _ TRUE _ _ _ _ _ _ _ _ _ _ _ _ _ _] -> w182
          tunnel: [w620 w625 w633 w639 w645 w650 w657 w664 w670 w673 w685 w697 w701 w711 w716 w720 w726 w736 w743 w748 w765 w774 w776 w782 w788 w799 w820 w826 w833 w838 w842 w850] -> w181
          tunnel: w178 -> [w619 w624 w632 w638 w644 w649 w656 w663 w669 w675 w684 w696 w703 w710 w718 w722 w725 w735 w745 w750 w755 w773 w780 w784 w795 w806 w822 w832 w836 w841 w846 w853]
          tunnel: [w619 w624 w632 w638 w644 w649 w656 w663 w669 w675 w683 w696 w703 w709 w718 w722 w725 w735 w745 w750 w754 w773 w780 w784 w795 w806 w822 w832 w836 w841 w846 w853] -> w177
          tunnel: [_ _ 0.4 ("Speed") -0.3 ("Speed") 0.19999999999999998 ("Speed") -0.2 ("Speed") _ 0.3 ("Speed") -0.5 ("Speed") _ _ _ _ 0.0 ("Speed") _ _ _ _ _ _ _ _ _ _ _ _ _ _ _ _ _ _] -> w175
          tunnel: [_ _ MOTOR_CONTROL_NO_PID_Type_Def."Front Back" ("Direction") _ MOTOR_CONTROL_NO_PID_Type_Def."Rotate" ("Direction") _ MOTOR_CONTROL_NO_PID_Type_Def."Stop" ("Direction") MOTOR_CONTROL_NO_PID_Type_Def."Left Right" ("Direction") MOTOR_CONTROL_NO_PID_Type_Def."Front Back" ("Direction") _ MOTOR_CONTROL_NO_PID_Type_Def."Latch" ("Direction") MOTOR_CONTROL_NO_PID_Type_Def."Latch" ("Direction") _ _ _ _ _ MOTOR_CONTROL_NO_PID_Type_Def."Latch" ("Direction") _ MOTOR_CONTROL_NO_PID_Type_Def."Init" ("Direction") _ MOTOR_CONTROL_NO_PID_Type_Def."Init" ("Direction") _ _ MOTOR_CONTROL_NO_PID_Type_Def."Latch" ("Direction") MOTOR_CONTROL_NO_PID_Type_Def."Latch" ("Direction") _ MOTOR_CONTROL_NO_PID_Type_Def."Latch" ("Direction") _ _ _ _] -> w173
          tunnel: [_ _ navX_type_def."Read Values" ("Mode") navX_type_def."Read Values" ("Mode") _ _ navX_type_def."Read Values" ("Mode") navX_type_def."Read Values" ("Mode") _ _ navX_type_def."Read Values" ("Mode") navX_type_def."Read Values" ("Mode") _ navX_type_def."Zero Yaw" ("Mode") _ _ navX_type_def."Zero Yaw" ("Mode") navX_type_def."Read Values" ("Mode") _ _ _ navX_type_def."Zero Yaw" ("Mode") _ _ navX_type_def."Read Values" ("Mode") navX_type_def."Read Values" ("Mode") _ navX_type_def."Read Values" ("Mode") _ _ _ _] -> w167
          tunnel: [_ _ _ _ _ _ _ _ _ _ _ I2C_MASTER_WRITE_NEW_Type_Def."Ultrasonic sensors" ("Arduino mode") _ _ I2C_MASTER_WRITE_NEW_Type_Def."Ultrasonic sensors" ("Arduino mode") _ _ _ _ _ _ _ I2C_MASTER_WRITE_NEW_Type_Def."Soft Reset" ("Arduino mode") _ _ _ _ _ _ I2C_MASTER_WRITE_NEW_Type_Def."Close Claw" ("Arduino mode") I2C_MASTER_WRITE_NEW_Type_Def."Open Claw" ("Arduino mode") I2C_MASTER_WRITE_NEW_Type_Def."zStepper 10k" ("Arduino mode")] -> w164
          tunnel: [_ _ _ _ _ _ _ _ _ _ _ _ _ _ _ _ _ TRUE ("Latch") _ _ _ _ _ _ _ _ _ _ _ _ _ FALSE ("Latch")] -> w163
          tunnel: [_ _ _ _ _ _ _ _ _ _ _ _ _ _ _ _ _ u8 0 ("y Stepper value") _ _ _ _ _ _ _ _ _ _ _ _ _ _] -> w162
          tunnel: w161 -> [_ _ _ _ _ _ _ _ _ _ _ _ _ _ _ _ _ _ _ _ _ _ _ _ _ _ w815 _ _ _ _ _]
          tunnel: w160 -> [_ _ _ _ _ _ _ _ _ _ _ _ _ _ _ _ _ _ _ _ _ _ _ _ _ _ w814 _ _ _ _ _]
          tunnel: w159 -> [w618 w623 w628 w635 w641 w647 w652 w659 w666 w672 w676 w687 w700 w704 w715 w719 w723 w730 w742 w746 w760 w769 w779 w781 w785 w796 w813 w823 w835 w840 w845 w852]
          tunnel: [w618 w623 w628 w635 w641 w647 w652 w659 w666 w672 w676 w687 w700 w704 w715 w719 w723 w730 w742 w746 w759 w769 w779 w781 w785 w796 w807 w823 w835 w840 w845 w852] -> w158
          frame "Exit" {
          }
          frame "----Movement States----" {
          }
          frame "FORWARD" {
          }
          frame "LEFT" {
            (unwired) I2C_MASTER_Type_Def."Last State" ("Arduino Mode")
          }
          frame "R-ACW" {
            (unwired) I2C_MASTER_Type_Def."Last State" ("Arduino Mode")
          }
          frame "R-CW" {
            (unwired) I2C_MASTER_Type_Def."Last State" ("Arduino Mode")
          }
          frame "STOP" {
            (unwired) I2C_MASTER_Type_Def."Last State" ("Arduino Mode")
            n59 = Wait (ms)(milliseconds to wait=u32 200) -> ()  [unwired: 1 out]
          }
          frame "RIGHT" {
            (unwired) I2C_MASTER_Type_Def."Last State" ("Arduino Mode")
          }
          frame "REVERSE" {
            (unwired) I2C_MASTER_Type_Def."Last State" ("Arduino Mode")
          }
          frame "----SENSOR READING---- " {
            (unwired) I2C_MASTER_Type_Def."Last State" ("Arduino Mode")
          }
          frame "READ ENCODERS" {
            (unwired) I2C_MASTER_Type_Def."Last State" ("Arduino Mode")
            # ">>> Current encoder distance >>>"
            # ">>> Ultrasonic Sensors Detect >>>"
            n60 = local read "Speed & distance"() -> (w682:T9)
            n61 = Unbundle By Name(w682) -> ("xDistance"=w681:dbl, "yDistance"=w680:dbl, "wDistance"=w679:dbl)
            n62 = Bundle By Name(cluster=w684, "xDistance"=w681, "yDistance"=w680, "wDistance"=w679) -> (w683:T16)
          }
          frame "ULTRASONIC READ" {
            # "Object detection"
            n63 = local read "Arduino Data"() -> (w693:T3)
            n64 = Unbundle By Name(w693) -> ("PING A"=w692:u8, "PING B"=w691:u8, "PING C"=w690:u8, "PING D"=w689:u8)
            n65 = Bundle By Name(cluster=w698, "PING_A"=w692, "PING_B"=w691, "PING_C"=w690, "PING_D"=w689) -> (w699:T15)
          }
          frame "----SYSTEM MODES----" {
            (unwired) I2C_MASTER_Type_Def."Last State" ("Arduino Mode")
          }
          frame "INIT" {
            (unwired) I2C_MASTER_Type_Def."Last State" ("Arduino Mode")
            w706 = 0
            w708 = 0.0
            # ">>State Logic  >>"
            n66 = Bundle By Name(cluster=w712, "PING_A"=w706, "PING_B"=w706, "PING_C"=w706, "PING_D"=w706) -> (w713:T15)
            n67 = Bundle By Name(cluster=w710, "xDistance"=w708, "yDistance"=w708, "wDistance"=w708) -> (w709:T16)
          }
          frame "ARDUINO MODE 0" {
          }
          frame "ARDUINO MODE 1" {
            (unwired) I2C_MASTER_Type_Def."Mode 1" ("Arduino Mode")
          }
          frame "NAVX CALIBRATE" {
            (unwired) I2C_MASTER_Type_Def."Last State" ("Arduino Mode")
            # "Adds a 15 second delay to the startup process \nfor the NavX to calibrate"
            n68 = Wait (ms)(milliseconds to wait=u32 5000) -> ()  [unwired: 1 out]
          }
          frame "NO ACTION", Default {
            n69 = case shown="4" w736 {
              tunnel: [0 100] -> w738
              frame 1, Default {
              }
              frame 4 {
              }
            }
          }
          frame "----RESET CASES----" {
            (unwired) I2C_MASTER_Type_Def."Last State" ("Arduino Mode")
          }
          frame "RESET ENCODERS" {
            (unwired) I2C_MASTER_Type_Def."Last State" ("Arduino Mode")
          }
          frame "RESET FLAGS" {
            (unwired) I2C_MASTER_Type_Def."Last State" ("Arduino Mode")
            # "Resets any software variables\nand/or non-critical states"
            n70 = Wait (ms)(milliseconds to wait=u32 20) -> ()  [unwired: 1 out]
            n71 = Bundle By Name(cluster=w755, "xDistance"=0.0, "yDistance"=0.0, "wDistance"=0.0) -> (w754:T16)
            n72 = Bundle By Name(cluster=w760, "Recognized Object"=FALSE, "Object X coordinate"=0.0, "Object Y coordinate"=0.0) -> (w759:T14)
            n73 = Bundle By Name(cluster=w767, "PING_A"=u8 0, "PING_B"=u8 0, "PING_C"=u8 0, "PING_D"=u8 0) -> (w766:T15)
          }
          frame "RESET YAW" {
            (unwired) I2C_MASTER_Type_Def."Last State" ("Arduino Mode")
            n74 = Wait (ms)(milliseconds to wait=u32 100) -> ()  [unwired: 1 out]
          }
          frame "RESET ARM" {
          }
          frame "--------CAM STATES-------" {
          }
          frame "OPEN LOG CAM" {
            n75 = call "Low-Level Grab.vi"("States"=State_control."Initialise", "Session In"=T23 "cam0") -> ("error out"=w790:errorcluster, "Session Out"=w791:T23)  [unwired: 7 in, 1 out]
            n76 = call "Low-Level Grab.vi"("error in (no error)"=w790, "States"=State_control."Start camera", "Session In"=w791) -> ()  [unwired: 6 in, 3 out]
          }
          frame "OPEN LIFE CAM" {
            n77 = call "Low-Level Grab.vi"("States"=State_control."Initialise", "Session In"=T23 "cam1") -> ("error out"=w801:errorcluster, "Session Out"=w802:T23)  [unwired: 7 in, 1 out]
            n78 = call "Low-Level Grab.vi"("error in (no error)"=w801, "States"=State_control."Start camera", "Session In"=w802) -> ()  [unwired: 6 in, 3 out]
          }
          frame "CAM ACQ" {
            n79 = call "Low-Level Grab.vi"("error in (no error)"=w814, "States"=State_control."Continuous Acquisition ") -> ("error out"=w817:errorcluster, "Image Out"=w818:T26)  [unwired: 7 in, 1 out]
            n80 = call "Object Detection SubVI.vi"("Error In"=w817, "Mode"="Mode", "Image Dest"=w815, "Image in"=w818) -> ("Object Center Coordinates"=w812:cluster{"x":sgl, "y":sgl}, "Object detection cluster"=w809:T2)  [unwired: 2 out]
            "Object detection cluster" <- w809
            "Object Center Coordinates" <- w812
            n81 = Unbundle By Name(w809) -> ("Object detected?"=w808:bool)
            n82 = Unbundle By Name(w812) -> ("x"=w811:sgl, "y"=w810:sgl)
            n83 = Bundle By Name(cluster=w813, "Recognized Object"=w808, "Object X coordinate"=w811, "Object Y coordinate"=w810) -> (w807:T14)
          }
          frame "CAM CLOSE" {
            n84 = call "Low-Level Grab.vi"("States"=State_control."Stop camera") -> ("error out"=w828:errorcluster, "Session Out"=w829:T23)  [unwired: 8 in, 1 out]
            n85 = call "Low-Level Grab.vi"("error in (no error)"=w828, "States"=State_control."Dispose all", "Session In"=w829) -> ()  [unwired: 6 in, 3 out]
          }
          frame "-----ARM ACTIONS-----" {
          }
          frame "CLOSE CLAW" {
          }
          frame "OPEN CLAW" {
          }
          frame "Z STEPPER CAM HEIGHT  " {
            n86 = Wait (ms)(milliseconds to wait=u32 500) -> ()  [unwired: 1 out]
          }
        }
        "State Logic" <- w181
        n87 = call "navX reading VI.vi"("Mode"=w167) -> ("NavX Readings"=w168:T8, "Status"=→"Status":T7)  [unwired: 2 in, 2 out]
        "NavX Readings" <- w168
        n88 = Unbundle By Name(w168) -> ("Yaw"=w166:dbl)
        n89 = local write "Arduino mode"(w164) -> ()
        n90 = local write "y Stepper value"(w162) -> ()
        n91 = local write "Latch"(w163) -> ()
        n92 = local read "TASK ENABLE"() -> (w172:bool)
        n93 = call "Motor Control NO PID.vi"("Yaw"=w166, "Speed"=w175, "Direction"=w173) -> ("Speed & distance"=→"Speed & distance":T9)  [unwired: 1 in, 1 out]
        n94 = Not(x=w172) -> (.not. x?=w171:bool)
        n95 = case shown="True" w182 {
          tunnel: w186 -> [w205 w225]
          tunnel: w190 -> [w201 w227]
          tunnel: [w205 w225] -> w195
          tunnel: [w201 w228] -> w194
          tunnel: w191 -> [_ w223]
          tunnel: w193 -> [_ w224]
          tunnel: w188 -> [w204 w230]
          tunnel: [w204 w230] -> w187
          tunnel: "STOP TASK" -> [_ w213]
          tunnel: w181 -> [w203 w229]
          tunnel: [w203 w226] -> w180
          tunnel: w177 -> [w202 w219]
          tunnel: [w202 w219] -> w176
          tunnel: w171 -> [_ w214]
          tunnel: [w200 w211] -> w170
          tunnel: w169 -> [w200 w210]
          tunnel: w158 -> [w199 w207]
          tunnel: [w199 w207] -> w157
          frame False {
          }
          frame True {
            # ">>Action Queue>>"
            # ">>State Logic Queue Reference >>"
            n96 = Or(x=w213, y=w214) -> (x .or. y?=w212:bool)
            n97 = Unbundle By Name(w207) -> ("Recognized Object"=w206:bool, "Object X coordinate"=w209:dbl, "Object Y coordinate"=w208:dbl)
            n98 = Unbundle By Name(w219) -> ("xDistance"=w216:dbl, "yDistance"=w217:dbl, "wDistance"=w218:dbl)
            n99 = Unbundle By Name(w230) -> ("PING_A"=w222:u8, "PING_B"=w221:u8, "PING_C"=w220:u8, "PING_D"=w215:u8)
            n100 = case shown="4, Default" w229 {
              tunnel: [w232 w235 w246 w253 w305 w317 w353 w399 w443 w500 w537 w587] -> w228
              tunnel: w227 -> [w232 w238 w247 w256 w307 w318 w354 w400 w449 w493 w541 w582]
              tunnel: [State_Type_Definitions,_for_0.26g_versions_and_later_2."Idle" ("Enum") State_Type_Definitions,_for_0.26g_versions_and_later_2."Idle" ("Enum") w242 w255 State_Type_Definitions,_for_0.26g_versions_and_later_2."Shutdown" ("Enum") w319 w356 w398 w444 w499 w538 w588] -> w226
              tunnel: w225 -> [_ _ w245 w259 _ w324 w366 w407 w448 w497 w542 w585]
              tunnel: w224 -> [_ _ _ w258 _ w323 w365 w406 w447 w496 w534 w584]
              tunnel: w223 -> [_ _ w244 w254 _ w322 w364 w405 w446 w495 w533 w583]
              tunnel: w212 -> [_ _ _ _ _ w316 w355 w402 w442 w498 w539 w586]
              tunnel: w222 -> [_ _ _ _ _ _ _ _ _ _ _ _]
              tunnel: w221 -> [_ _ _ _ _ _ w362 _ w440 w488 w544 _]
              tunnel: w220 -> [_ _ _ _ _ _ w361 _ w441 w489 w543 _]
              tunnel: w218 -> [_ _ _ _ _ _ _ w404 _ _ _ _]
              tunnel: w217 -> [_ _ _ _ _ w315 _ _ _ _ _ _]
              tunnel: w216 -> [_ _ _ _ _ _ _ _ _ w484 _ _]
              tunnel: w215 -> [_ _ _ _ _ _ _ _ _ _ _ _]
              tunnel: [State_Type_Definitions,_for_0.26g_versions_and_later_2."Idle" ("Enum") State_Type_Definitions,_for_0.26g_versions_and_later_2."Idle" ("Enum") State_Type_Definitions,_for_0.26g_versions_and_later_2."Idle" ("Enum") State_Type_Definitions,_for_0.26g_versions_and_later_2."Idle" ("Enum") State_Type_Definitions,_for_0.26g_versions_and_later_2."Shutdown" ("Enum") w312 w352 w395 w435 w483 w536 w589] -> w211
              tunnel: w210 -> [_ _ w242 _ _ _ _ _ _ _ _ _]
              tunnel: w206 -> [_ _ _ _ _ _ _ _ _ _ _ w581]
              tunnel: w209 -> [_ _ _ _ _ _ _ _ _ _ _ _]
              tunnel: w208 -> [_ _ _ _ _ _ _ _ _ _ _ _]
              frame 0 {
              }
              frame 1 {
                n101 = for {
                  shift-right: [w241] -> w235
                  shift-left: w238 -> [w240]
                  tunnel: string[] ["INIT", "NAVX CALIBRATE", "RESET FLAGS", "RESET YAW", "RESET ARM"] -> [w239] mode=indexing
                  n102 = Enqueue Element(queue=w240, element=w239) -> (queue out=w241:refnum<queue>)  [unwired: 2 in, 2 out]
                }
              }
              frame 3 {
                n103 = Flush Queue(queue=w245, error in (no error)=w244) -> ()  [unwired: 3 out]
                n104 = for {
                  shift-right: [w251] -> w246
                  shift-left: w247 -> [w250]
                  tunnel: string[] ["STOP", "RESET ENCODERS", "RESET YAW", "ARDUINO MODE 0", "CAM CLOSE", "RESET ARM"] -> [w249] mode=indexing
                  n105 = Enqueue Element(queue=w250, element=w249) -> (queue out=w251:refnum<queue>)  [unwired: 2 in, 2 out]
                }
              }
              frame 4, Default {
                (unwired) TRUE ("Green LED")
                n106 = Dequeue Element(queue=w259, timeout in ms (-1)=w258, error in (no error)=w254) -> (element=w257:T11)  [unwired: 3 out]
                n107 = case shown="\"Start Task 6\"" w257 {
                  tunnel: [w261 w268 w275 w282 w289 w296 w298] -> w253
                  tunnel: w256 -> [w262 w269 w276 w283 w290 w296 w299]
                  tunnel: [State_Type_Definitions."Task 1" ("Enum") State_Type_Definitions."Task 2" ("Enum") State_Type_Definitions,_for_0.26g_versions_and_later_2."Task 3" ("Enum") State_Type_Definitions,_for_0.26g_versions_and_later_2."Task 4_A" ("Enum") State_Type_Definitions."Task 6" ("Enum") State_Type_Definitions,_for_0.26g_versions_and_later_2."Idle" ("Enum") State_Type_Definitions,_for_0.26g_versions_and_later_2."Shutdown" ("Enum")] -> w255
                  frame "Start Task 1" {
                    n108 = for {
                      shift-right: [w266] -> w261
                      shift-left: w262 -> [w265]
                      tunnel: string[] ["RESET ENCODERS", "RESET YAW", "FORWARD", "READ ENCODERS"] -> [w264] mode=indexing
                      n109 = Enqueue Element(queue=w265, element=w264) -> (queue out=w266:refnum<queue>)  [unwired: 2 in, 2 out]
                    }
                  }
                  frame "Start Task 2" {
                    n110 = for {
                      shift-right: [w273] -> w268
                      shift-left: w269 -> [w272]
                      tunnel: string[] ["RESET ENCODERS", "RESET YAW", "ULTRASONIC READ", "ARDUINO MODE 0"] -> [w271] mode=indexing
                      n111 = Enqueue Element(queue=w272, element=w271) -> (queue out=w273:refnum<queue>)  [unwired: 2 in, 2 out]
                    }
                  }
                  frame "Start Task 3" {
                    n112 = for {
                      shift-right: [w280] -> w275
                      shift-left: w276 -> [w279]
                      tunnel: string[] ["RESET ENCODERS", "READ ENCODERS", "R-ACW"] -> [w278] mode=indexing
                      n113 = Enqueue Element(queue=w279, element=w278) -> (queue out=w280:refnum<queue>)  [unwired: 2 in, 2 out]
                    }
                  }
                  frame "Start Task 4" {
                    n114 = for {
                      shift-right: [w287] -> w282
                      shift-left: w283 -> [w286]
                      tunnel: string[] ["STOP", "RESET YAW", "RESET ENCODERS", "ARDUINO MODE 0", "ULTRASONIC READ", "FORWARD"] -> [w285] mode=indexing
                      n115 = Enqueue Element(queue=w286, element=w285) -> (queue out=w287:refnum<queue>)  [unwired: 2 in, 2 out]
                    }
                  }
                  frame "Start Task 6" {
                    n116 = for {
                      shift-right: [w294] -> w289
                      shift-left: w290 -> [w293]
                      tunnel: string[] ["OPEN LOG CAM", "CAM ACQ", "RESET YAW", "Z STEPPER CAM HEIGHT", "", ""] -> [w292] mode=indexing
                      n117 = Enqueue Element(queue=w293, element=w292) -> (queue out=w294:refnum<queue>)  [unwired: 2 in, 2 out]
                    }
                  }
                  frame "None", Default {
                  }
                  frame "Exit" {
                    n118 = for {
                      shift-right: [w303] -> w298
                      shift-left: w299 -> [w302]
                      tunnel: string[] ["STOP", "RESET ENCODERS", "RESET YAW", "EXIT"] -> [w301] mode=indexing
                      n119 = Enqueue Element(queue=w302, element=w301) -> (queue out=w303:refnum<queue>)  [unwired: 2 in, 2 out]
                    }
                  }
                }
              }
              frame 5 {
                n120 = for {
                  shift-right: [w311] -> w305
                  shift-left: w307 -> [w310]
                  tunnel: string[] ["INIT", "RESET ENCODERS", "RESET FLAGS", "EXIT"] -> [w309] mode=indexing
                  n121 = Enqueue Element(queue=w310, element=w309) -> (queue out=w311:refnum<queue>)  [unwired: 2 in, 2 out]
                }
              }
              frame 6 {
                # "Use 250"
                n122 = Dequeue Element(queue=w324, timeout in ms (-1)=w323, error in (no error)=w322) -> (element=w321:T11)  [unwired: 3 out]
                n123 = Greater?(x=w315, y=250.0) -> (0:w313:bool)
                n124 = Or(x=w313, y=w316) -> (x .or. y?=w320:bool)
                n125 = case shown="\"None\", Default" w321 {
                  tunnel: w320 -> [w327 _]
                  tunnel: [w331 State_Type_Definitions,_for_0.26g_versions_and_later_2."True Stop" ("Enum")] -> w319
                  tunnel: w318 -> [w328 w346]
                  tunnel: [w326 w345] -> w317
                  tunnel: [State_Type_Definitions,_for_0.26g_versions_and_later_2."Idle" ("Enum") State_Type_Definitions,_for_0.26g_versions_and_later_2."Shutdown" ("Enum")] -> w312
                  frame "None", Default {
                    n126 = case shown="True" w327 {
                      tunnel: w328 -> [w334 w340]
                      tunnel: [w333 w338] -> w326
                      frame False {
                        n127 = for {
                          shift-right: [w336] -> w333
                          shift-left: w334 -> [w337]
                          tunnel: string[] ["READ ENCODERS", "FORWARD"] ("element") -> [w335] mode=indexing
                          n128 = Enqueue Element(queue=w337, element=w335) -> (queue out=w336:refnum<queue>)  [unwired: 2 in, 2 out]
                        }
                      }
                      frame True {
                        n129 = for {
                          shift-right: [w342] -> w338
                          shift-left: w340 -> [w343]
                          tunnel: string[] ["RESET YAW", "RESET ENCODERS", "STOP", "ARDUINO MODE 0"] -> [w341] mode=indexing
                          n130 = Enqueue Element(queue=w343, element=w341) -> (queue out=w342:refnum<queue>)  [unwired: 2 in, 2 out]
                        }
                      }
                    }
                    n131 = Select(t=State_Type_Definitions,_for_0.26g_versions_and_later_2."True Stop" ("Enum"), s=w327, f=State_Type_Definitions."Task 1" ("Enum")) -> (s? t:f=w331:u16)
                  }
                  frame "Exit" {
                    n132 = for {
                      shift-right: [w350] -> w345
                      shift-left: w346 -> [w351]
                      tunnel: string[] ["STOP", "RESET ENCODERS", "RESET YAW", ""] -> [w349] mode=indexing
                      n133 = Enqueue Element(queue=w351, element=w349) -> (queue out=w350:refnum<queue>)  [unwired: 2 in, 2 out]
                    }
                  }
                }
              }
              frame 7 {
                w360 = u16 10 ("y")
                # ">>Object detected>>"
                n134 = Dequeue Element(queue=w366, timeout in ms (-1)=w365, error in (no error)=w364) -> (element=w363:T11)  [unwired: 3 out]
                n135 = Less?(x=w362, y=w360) -> (x < y?=w359:bool)
                n136 = Less?(x=w361, y=w360) -> (x < y?=w358:bool)
                n137 = Or(x=w359, y=w358) -> (x .or. y?=w357:bool)
                "Object detected?" <- w357
                n138 = case shown="\"None\", Default" w363 {
                  tunnel: w357 -> [w370 _]
                  tunnel: [w372 State_Type_Definitions,_for_0.26g_versions_and_later_2."True Stop" ("Enum")] -> w356
                  tunnel: w355 -> [w371 _]
                  tunnel: w354 -> [w369 w389]
                  tunnel: [w368 w390] -> w353
                  tunnel: [State_Type_Definitions,_for_0.26g_versions_and_later_2."Idle" ("Enum") State_Type_Definitions,_for_0.26g_versions_and_later_2."Shutdown" ("Enum")] -> w352
                  frame "None", Default {
                    n139 = case shown="True" w370 {
                      tunnel: w369 -> [w376 w383]
                      tunnel: [w377 w382] -> w368
                      frame False {
                        n140 = for {
                          tunnel: string[] ["ULTRASONIC READ", "STOP"] ("element") -> [w378] mode=indexing
                          shift-right: [w380] -> w377
                          shift-left: w376 -> [w379]
                          n141 = Enqueue Element(queue=w379, element=w378) -> (queue out=w380:refnum<queue>)  [unwired: 2 in, 2 out]
                        }
                      }
                      frame True {
                        n142 = for {
                          shift-right: [w385] -> w382
                          shift-left: w383 -> [w386]
                          tunnel: string[] ["REVERSE", "ULTRASONIC READ"] -> [w384] mode=indexing
                          n143 = Enqueue Element(queue=w386, element=w384) -> (queue out=w385:refnum<queue>)  [unwired: 2 in, 2 out]
                        }
                      }
                    }
                    n144 = Select(t=State_Type_Definitions,_for_0.26g_versions_and_later_2."True Stop" ("Enum"), s=w371, f=State_Type_Definitions."Task 2" ("Enum")) -> (s? t:f=w372:u16)
                  }
                  frame "Exit" {
                    n145 = for {
                      shift-right: [w393] -> w390
                      shift-left: w389 -> [w394]
                      tunnel: string[] ["STOP", "RESET ENCODERS", "RESET YAW", "ARDUINO MODE 0"] -> [w392] mode=indexing
                      n146 = Enqueue Element(queue=w394, element=w392) -> (queue out=w393:refnum<queue>)  [unwired: 2 in, 2 out]
                    }
                  }
                }
              }
              frame 10 {
                n147 = Dequeue Element(queue=w407, timeout in ms (-1)=w406, error in (no error)=w405) -> (element=w396:T11)  [unwired: 3 out]
                n148 = Greater?(x=w404, y=150.0) -> (0:w401:bool)
                n149 = Or(x=w401, y=w402) -> (x .or. y?=w397:bool)
                n150 = case shown="\"Exit\"" w396 {
                  tunnel: w397 -> [w410 _]
                  tunnel: [w414 State_Type_Definitions,_for_0.26g_versions_and_later_2."True Stop" ("Enum")] -> w398
                  tunnel: w400 -> [w411 w430]
                  tunnel: [w409 w429] -> w399
                  tunnel: [State_Type_Definitions,_for_0.26g_versions_and_later_2."Idle" ("Enum") State_Type_Definitions,_for_0.26g_versions_and_later_2."Shutdown" ("Enum")] -> w395
                  frame "None", Default {
                    n151 = case shown="False" w410 {
                      tunnel: w411 -> [w417 w423]
                      tunnel: [w416 w421] -> w409
                      frame False {
                        n152 = for {
                          shift-right: [w419] -> w416
                          shift-left: w417 -> [w420]
                          tunnel: string[] ["READ ENCODERS", "R-ACW"] ("element") -> [w418] mode=indexing
                          n153 = Enqueue Element(queue=w420, element=w418) -> (queue out=w419:refnum<queue>)  [unwired: 2 in, 2 out]
                        }
                      }
                      frame True {
                        n154 = for {
                          shift-right: [w425] -> w421
                          shift-left: w423 -> [w426]
                          tunnel: string[] ["RESET YAW", "RESET ENCODERS", "STOP", "ARDUINO MODE 0"] -> [w424] mode=indexing
                          n155 = Enqueue Element(queue=w426, element=w424) -> (queue out=w425:refnum<queue>)  [unwired: 2 in, 2 out]
                        }
                      }
                    }
                    n156 = Select(t=State_Type_Definitions,_for_0.26g_versions_and_later_2."True Stop" ("Enum"), s=w410, f=State_Type_Definitions,_for_0.26g_versions_and_later_2."Task 3" ("Enum")) -> (s? t:f=w414:T10)
                  }
                  frame "Exit" {
                    n157 = for {
                      shift-right: [w433] -> w429
                      shift-left: w430 -> [w434]
                      tunnel: string[] ["STOP", "RESET ENCODERS", "RESET YAW", ""] -> [w432] mode=indexing
                      n158 = Enqueue Element(queue=w434, element=w432) -> (queue out=w433:refnum<queue>)  [unwired: 2 in, 2 out]
                    }
                  }
                }
              }
              frame 11 {
                w439 = 20
                # ">> Outputs true if object detected >>"
                # ">> Manual override >>"
                n159 = Dequeue Element(queue=w448, timeout in ms (-1)=w447, error in (no error)=w446) -> (element=w445:T11)  [unwired: 3 out]
                n160 = Less?(x=w441, y=w439) -> (x < y?=w437:bool)
                n161 = Less?(x=w440, y=w439) -> (x < y?=w438:bool)
                n162 = And(x=w438, y=w437) -> (x .and. y?=w436:bool)
                "Detect?" <- w436
                n163 = case shown="\"None\", Default" w445 {
                  tunnel: [w458 State_Type_Definitions,_for_0.26g_versions_and_later_2."True Stop" ("Enum")] -> w444
                  tunnel: [w456 w477] -> w443
                  tunnel: w449 -> [w455 _]
                  tunnel: w442 -> [w453 _]
                  tunnel: w436 -> [w451 _]
                  tunnel: [w450 State_Type_Definitions,_for_0.26g_versions_and_later_2."Shutdown" ("Enum")] -> w435
                  frame "None", Default {
                    # ">> WIill proceed to part ii if not manual override >>"
                    # ">>If ENABLE or Trigger is set to true>>"
                    n164 = Or(x=w451, y=w453) -> (x .or. y?=w452:bool)
                    n165 = case shown="False" w452 {
                      tunnel: [w465 w470] -> w456
                      tunnel: w455 -> [w463 w469]
                      frame False {
                        n166 = for {
                          shift-right: [w467] -> w465
                          shift-left: w463 -> [w468]
                          tunnel: string[] ["FORWARD", "ULTRASONIC READ", ""] ("element") -> [w466] mode=indexing
                          n167 = Enqueue Element(queue=w468, element=w466) -> (queue out=w467:refnum<queue>)  [unwired: 2 in, 2 out]
                        }
                      }
                      frame True {
                        n168 = for {
                          shift-right: [w473] -> w470
                          shift-left: w469 -> [w474]
                          tunnel: string[] ["STOP", "RESET ENCODERS", "RESET YAW", "ARDUINO MODE 0"] -> [w472] mode=indexing
                          n169 = Enqueue Element(queue=w474, element=w472) -> (queue out=w473:refnum<queue>)  [unwired: 2 in, 2 out]
                        }
                      }
                    }
                    n170 = case shown="False" w453 {
                      tunnel: [State_Type_Definitions,_for_0.26g_versions_and_later_2."True Stop" ("Enum") State_Type_Definitions,_for_0.26g_versions_and_later_2."True Stop" ("Enum")] -> w454
                      tunnel: [State_Type_Definitions,_for_0.26g_versions_and_later_2."Task 4_B" ("Enum") State_Type_Definitions,_for_0.26g_versions_and_later_2."Idle" ("Enum")] -> w450
                      frame False {
                      }
                      frame True {
                      }
                    }
                    n171 = Select(t=w454, s=w452, f=State_Type_Definitions,_for_0.26g_versions_and_later_2."Task 4_A" ("Enum")) -> (s? t:f=w458:T10)
                  }
                  frame "Exit" {
                    n172 = for {
                      shift-right: [w480] -> w477
                      shift-left: _ -> [w481]
                      tunnel: string[] ["STOP", "RESET ENCODERS", "RESET YAW", ""] -> [w479] mode=indexing
                      n173 = Enqueue Element(queue=w481, element=w479) -> (queue out=w480:refnum<queue>)  [unwired: 2 in, 2 out]
                    }
                  }
                }
              }
              frame 12 {
                w492 = 20
                # ">> Outputs true if 150 mm has been moved >>"
                # ">> Outputs true if sensor not obstructed>>"
                # ">> Manual override >>"
                n174 = Dequeue Element(queue=w497, timeout in ms (-1)=w496, error in (no error)=w495) -> (element=w494:T11)  [unwired: 3 out]
                n175 = Greater?(x=w489, y=w492) -> (0:w490:bool)
                n176 = Greater?(x=w488, y=w492) -> (0:w491:bool)
                n177 = Greater Or Equal?(x=w484, y=80.0) -> (x >= y?=w486:bool)
                n178 = And(x=w491, y=w490) -> (x .and. y?=w485:bool)
                n179 = And(x=w486, y=w485) -> (x .and. y?=w482:bool)
                n180 = case shown="\"None\", Default" w494 {
                  tunnel: [w509 State_Type_Definitions,_for_0.26g_versions_and_later_2."True Stop" ("Enum")] -> w499
                  tunnel: [w507 w528] -> w500
                  tunnel: w493 -> [w506 _]
                  tunnel: w498 -> [w504 _]
                  tunnel: w482 -> [w502 _]
                  tunnel: [w501 State_Type_Definitions,_for_0.26g_versions_and_later_2."Shutdown" ("Enum")] -> w483
                  frame "None", Default {
                    # ">> WIill proceed to part ii if not manual override >>"
                    # ">>If ENABLE or Trigger is set to true>>"
                    n181 = Or(x=w502, y=w504) -> (x .or. y?=w503:bool)
                    n182 = case shown="False" w503 {
                      tunnel: [w516 w521] -> w507
                      tunnel: w506 -> [w514 w520]
                      frame False {
                        n183 = for {
                          shift-right: [w518] -> w516
                          shift-left: w514 -> [w519]
                          tunnel: string[] ["RIGHT", "ULTRASONIC READ", "READ ENCODERS"] ("element") -> [w517] mode=indexing
                          n184 = Enqueue Element(queue=w519, element=w517) -> (queue out=w518:refnum<queue>)  [unwired: 2 in, 2 out]
                        }
                      }
                      frame True {
                        n185 = for {
                          shift-right: [w524] -> w521
                          shift-left: w520 -> [w525]
                          tunnel: string[] ["STOP", "RESET ENCODERS", "RESET YAW", "ARDUINO MODE 0"] -> [w523] mode=indexing
                          n186 = Enqueue Element(queue=w525, element=w523) -> (queue out=w524:refnum<queue>)  [unwired: 2 in, 2 out]
                        }
                      }
                    }
                    n187 = case shown="True" w504 {
                      tunnel: [State_Type_Definitions,_for_0.26g_versions_and_later_2."True Stop" ("Enum") State_Type_Definitions,_for_0.26g_versions_and_later_2."True Stop" ("Enum")] -> w505
                      tunnel: [State_Type_Definitions,_for_0.26g_versions_and_later_2."Task 4_C" ("Enum") State_Type_Definitions,_for_0.26g_versions_and_later_2."Idle" ("Enum")] -> w501
                      frame False {
                      }
                      frame True {
                      }
                    }
                    n188 = Select(t=w505, s=w503, f=State_Type_Definitions,_for_0.26g_versions_and_later_2."Task 4_B" ("Enum")) -> (s? t:f=w509:T10)
                  }
                  frame "Exit" {
                    n189 = for {
                      shift-right: [w531] -> w528
                      shift-left: _ -> [w532]
                      tunnel: string[] ["STOP", "RESET ENCODERS", "RESET YAW", ""] -> [w530] mode=indexing
                      n190 = Enqueue Element(queue=w532, element=w530) -> (queue out=w531:refnum<queue>)  [unwired: 2 in, 2 out]
                    }
                  }
                }
              }
              frame 13 {
                w547 = 20
                # ">> Outputs true if object detected >>"
                # ">> Manual override >>"
                n191 = Dequeue Element(queue=w542, timeout in ms (-1)=w534, error in (no error)=w533) -> (element=w535:T11)  [unwired: 3 out]
                n192 = Less?(x=w543, y=w547) -> (x < y?=w545:bool)
                n193 = Less?(x=w544, y=w547) -> (x < y?=w546:bool)
                n194 = And(x=w546, y=w545) -> (x .and. y?=w540:bool)
                n195 = case shown="\"None\", Default" w535 {
                  tunnel: [w556 State_Type_Definitions,_for_0.26g_versions_and_later_2."True Stop" ("Enum")] -> w538
                  tunnel: [w554 w576] -> w537
                  tunnel: w541 -> [w553 w573]
                  tunnel: w539 -> [w551 _]
                  tunnel: w540 -> [w549 _]
                  tunnel: [w548 State_Type_Definitions,_for_0.26g_versions_and_later_2."Shutdown" ("Enum")] -> w536
                  frame "None", Default {
                    # ">> WIill proceed to part ii if not manual override >>"
                    # ">>If ENABLE or Trigger is set to true>>"
                    n196 = Or(x=w549, y=w551) -> (x .or. y?=w550:bool)
                    n197 = case shown="False" w550 {
                      tunnel: [w563 w568] -> w554
                      tunnel: w553 -> [w561 w567]
                      frame False {
                        n198 = for {
                          shift-right: [w565] -> w563
                          shift-left: w561 -> [w566]
                          tunnel: string[] ["FORWARD", "ULTRASONIC READ", ""] ("element") -> [w564] mode=indexing
                          n199 = Enqueue Element(queue=w566, element=w564) -> (queue out=w565:refnum<queue>)  [unwired: 2 in, 2 out]
                        }
                      }
                      frame True {
                        n200 = for {
                          shift-right: [w571] -> w568
                          shift-left: w567 -> [w572]
                          tunnel: string[] ["STOP", "RESET ENCODERS", "RESET YAW", "ARDUINO MODE 0"] -> [w570] mode=indexing
                          n201 = Enqueue Element(queue=w572, element=w570) -> (queue out=w571:refnum<queue>)  [unwired: 2 in, 2 out]
                        }
                      }
                    }
                    n202 = case shown="True" w551 {
                      tunnel: [State_Type_Definitions,_for_0.26g_versions_and_later_2."True Stop" ("Enum") State_Type_Definitions,_for_0.26g_versions_and_later_2."True Stop" ("Enum")] -> w552
                      tunnel: [State_Type_Definitions,_for_0.26g_versions_and_later_2."Idle" ("Enum") State_Type_Definitions,_for_0.26g_versions_and_later_2."Idle" ("Enum")] -> w548
                      frame False {
                      }
                      frame True {
                      }
                    }
                    n203 = Select(t=w552, s=w550, f=State_Type_Definitions,_for_0.26g_versions_and_later_2."Task 4_C" ("Enum")) -> (s? t:f=w556:T10)
                  }
                  frame "Exit" {
                    n204 = for {
                      shift-right: [w579] -> w576
                      shift-left: w573 -> [w580]
                      tunnel: string[] ["STOP", "RESET ENCODERS", "RESET YAW", ""] -> [w578] mode=indexing
                      n205 = Enqueue Element(queue=w580, element=w578) -> (queue out=w579:refnum<queue>)  [unwired: 2 in, 2 out]
                    }
                  }
                }
              }
              frame 13 {
                (unwired) u16 10 ("y")
                n206 = Dequeue Element(queue=w585, timeout in ms (-1)=w584, error in (no error)=w583) -> (element=w590:T11)  [unwired: 3 out]
                n207 = case shown="\"None\", Default" w590 {
                  tunnel: [w596 State_Type_Definitions,_for_0.26g_versions_and_later_2."True Stop" ("Enum")] -> w588
                  tunnel: [w595 w613] -> w587
                  tunnel: [State_Type_Definitions,_for_0.26g_versions_and_later_2."Idle" ("Enum") State_Type_Definitions,_for_0.26g_versions_and_later_2."Shutdown" ("Enum")] -> w589
                  tunnel: w586 -> [w593 _]
                  tunnel: w581 -> [w592 _]
                  tunnel: w582 -> [w591 _]
                  frame "None", Default {
                    n208 = case shown="True" w592 {
                      tunnel: [w601 w607] -> w595
                      tunnel: w591 -> [w599 w605]
                      frame False {
                        n209 = for {
                          tunnel: string[] ["CAM ACQ", "STOP"] ("element") -> [w602] mode=indexing
                          shift-right: [w604] -> w601
                          shift-left: w599 -> [w603]
                          n210 = Enqueue Element(queue=w603, element=w602) -> (queue out=w604:refnum<queue>)  [unwired: 2 in, 2 out]
                        }
                      }
                      frame True {
                        n211 = for {
                          shift-right: [w609] -> w607
                          shift-left: w605 -> [w610]
                          tunnel: string[] ["REVERSE", "CAM ACQ"] -> [w608] mode=indexing
                          n212 = Enqueue Element(queue=w610, element=w608) -> (queue out=w609:refnum<queue>)  [unwired: 2 in, 2 out]
                        }
                      }
                    }
                    n213 = Select(t=State_Type_Definitions,_for_0.26g_versions_and_later_2."True Stop" ("Enum"), s=w593, f=State_Type_Definitions."Task 6" ("Enum")) -> (s? t:f=w596:u16)
                  }
                  frame "Exit" {
                    n214 = for {
                      shift-right: [w616] -> w613
                      shift-left: _ -> [w617]
                      tunnel: string[] ["STOP", "RESET ENCODERS", "RESET YAW", "ARDUINO MODE 0"] -> [w615] mode=indexing
                      n215 = Enqueue Element(queue=w617, element=w615) -> (queue out=w616:refnum<queue>)  [unwired: 2 in, 2 out]
                    }
                  }
                }
              }
            }
          }
        }
      }
      n216 = call <vilib>:"DIO Close.vi"("error in (no error)"=w21, "DIO Info In"=w24) -> ()  [unwired: 9 in, 1 out]
      n217 = call <vilib>:"DIO Close.vi"("error in (no error)"=w31, "DIO Info In"=w33) -> ()  [unwired: 9 in, 1 out]
      n218 = call <vilib>:"NavX Close.vi"("error in (no error)"=w19, "NavX Info In"=w20) -> ()  [unwired: 9 in, 1 out]
      n219 = call <vilib>:"DIO Close.vi"("error in (no error)"=w26, "DIO Info In"=w28) -> ()  [unwired: 9 in, 1 out]
      n220 = call <vilib>:"DIO Close.vi"("error in (no error)"=w7, "DIO Info In"=w8) -> ()  [unwired: 9 in, 1 out]
      n221 = call <vilib>:"DIO Close.vi"("error in (no error)"=w2, "DIO Info In"=w3) -> ()  [unwired: 9 in, 1 out]
      n222 = while {
        stop <- w69 stop-if-true
        n223 = call <vilib>:"RT Get CPU Loads.vi"() -> ("CPU loads"=→"CPU loads":T1[])  [unwired: 10 in, 1 out]
        n224 = Wait (ms)(milliseconds to wait=u32 100) -> ()  [unwired: 1 out]
        n225 = call "FGV Bool.vi"("Init/Read/Write State"=States_for_Action_Engine."Read") -> ("Output node"=w69:bool)  [unwired: 2 in, 1 out]
      }
      n226 = Merge Errors "Merge Errors"(w61, w60) -> (w43:errorcluster)
      n227 = Merge Errors(w47, w43) -> (w42:errorcluster)
      n228 = Destroy User Event(user event=w64, error in=w42) -> ()  [unwired: 1 out]
      n229 = Destroy User Event(user event=w65, error in=w42) -> ()  [unwired: 1 out]
      n230 = Unregister For Events(event registration refnum=w56, error in=w42) -> ()  [unwired: 1 out]
      n231 = Release Queue(queue=w38, error in (no error)=w42) -> (error out=w18:errorcluster)  [unwired: 1 in, 2 out]
      n232 = Release Queue(queue=w55, error in (no error)=w42) -> ()  [unwired: 1 in, 3 out]
      n233 = call <vilib>:"Simple Error Handler.vi"("error in (no error)"=w18) -> ("error out"=w17:errorcluster)  [unwired: 4 in, 4 out]
      n234 = call <vilib>:"Reset myRIO.vi"("error in (no error)"=w17) -> ("error out"=→"error out":errorcluster)  [unwired: 10 in]
    }
    frame #2 {
      n235 = call "Imaq Dispose"("All Images? (No)"=TRUE) -> ()  [unwired: 5 in, 1 out]
      n236 = Wait (ms)(milliseconds to wait=u32 100) -> ()  [unwired: 1 out]
    }
  }
